vi "Uncaging Dual.vi"() -> ()   [LabVIEW 2012]
uses:
  Custom Controls and Typedefs/Calibrate_Button.ctl
  Custom Controls and Typedefs/SciScan System Information Cluster.ctl
  <vilib>/Utility/miscctls.llb/LVRowAndColumnTypeDef.ctl
  Custom Controls and Typedefs/LineScan settings Status.ctl
  Custom Controls and Typedefs/LineScan Image Status.ctl
  <vilib>/vision/Image Controls.llb/IMAQ Image.ctl
  <vilib>/Utility/miscctls.llb/LVRowAndColumnUnsignedTypeDef.ctl
  modules/hyperscope modules/hyperscope subVIs/Timebase and Trigger Routing.ctl
  Custom Controls/Image Types.ctl
  Custom Controls/scan mode main settings tab.ctl
  Custom Controls/MAIN Image panel reso tab Control type def.ctl
  Custom Controls/MAIN Image panel tab Control type def.ctl
  Custom Controls and Typedefs/SamplingRatesCluster.ctl
  Custom Controls and Typedefs/GroupParameters_Cluster.ctl
  Custom Controls and Typedefs/TriggerParameters_Cluster.ctl
  Custom Controls and Typedefs/UncageType.ctl
  GFG/GFG Translator Wrapper/GFGTranslator_Action.ctl
  GFG/GFG Translator Wrapper/GFGTranslator_Datatype.ctl
  GFG/GFG Translator Wrapper/GFGTranslator_errors.ctl
  GFG/GFGbooleanGet.vi
  GFG/GFGstringGet.vi
  save ROI.vi
  <vilib>/Utility/config.llb/Read Key (String).vi
  Global Variable_Waveforms.vi
  GFG/GFGfpRefGet.vi
  GFG/GFGpathGet.vi
  <vilib>/Utility/file.llb/Read From Spreadsheet File (string).vi
  GFG/GFG library.lvlib
  <vilib>/Utility/config.llb/NI_LVConfig.lvlib
panel:
  in  "Stimulation Protocol":enum32{"Protocol Editor", "Waveforms"}(tab)
  in  "Protocol Editor":i32[](listbox)
  in  "Enable/Disable All":bool=TRUE
  in  "Delete":bool
  in  "Reverse":bool
  in  "random":bool
  out "Waveform Graph":waveform(dbl)[](graph)
  out "StimModuleStatus":string caption="Status"
  in  "reset zoom_Photo-Stim_UI":bool
  out "Image1":T1(plugin-control)
  in  "Channel Selector":T2(tab)
  in  "Auto Update?":bool=TRUE
  out "Time for generating waveforms (ms)":u32
  in  "Update waveform and Timing":bool
  in  "Rep interval (s)":dbl=0.1 min=1.0 step=1.0
  in  "Pre-Stim Baseline":dbl
  in  "Pre-stim baseline (s)":bool
  in  "Group reps":dbl=1.0 min=1.0 step=1.0
  in  "Protocol Name":string="New_Stim_Protocol"
  in  "Load Stim Protocol":bool
  in  "Save Stim Protocol":bool
  in  "Columns":i32=6 min=1
  in  "Rows":i32=6 min=1
  in  "Y position":i32=128
  in  "X postition":i32=128
  in  "Grid spacing (µm)":dbl=10.0
  in  "GRID":bool
  in  "Spot repetitions":dbl=5.0 min=1.0 step=1.0
  in  "Stim duration (s)":dbl=0.0001 caption="(10u to 10m)" min=1e-05 max=0.01 step=1e-05 format="%#_6p"
  in  "Pre-stim settling time (s)":dbl=0.0008 caption="(800u to 1)" min=0.0008 max=1.0 format="%#_6p"
  in  "Stim interval (s)":dbl=0.00030000000000000003 caption="(300u to 1)" min=0.00030000000000000003 max=1.0 step=0.005 format="%#_6p"
  in  "Stim Power (%)":dbl(slide) min=0.0 max=100.0 step=0.1 scale=0.0..100.0
  out "Group Duration (s)":dbl
  in  "Uncage and Image":bool
  in  "Uncage ONLY":bool
  in  "stop":bool
  out "Total time (s)":dbl
  in  "Imaging Shutter":bool caption="Imaging Path Shutter"
  in  "Uncaging Shutter":bool caption="Stim Path Shutter"
  in  "Wait for external trigger":bool
  in  "Calibrate":T3
  # "General Stimulation Parameters"
  # "to zoom out press and hold Shift"
  # "Stimulation Protocol"
  # "Protocol Parameters"
  # "File Operations"
  # "Grid Parameters"
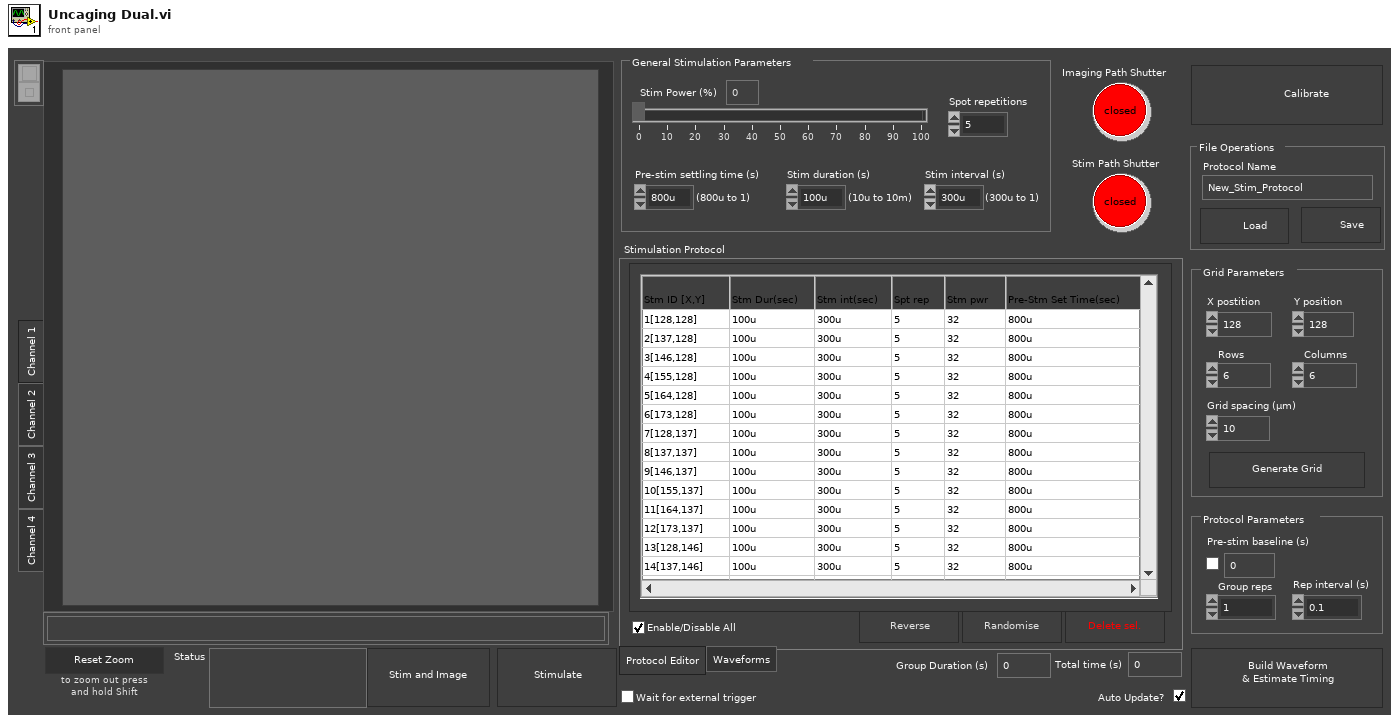
[diagram p1: front panel]
types:
  T1 = typedef "IMAQ Image.ctl" = refnum<image>
  T2 = enum32{"Channel 1", "Channel 2", "Channel 3", "Channel 4"}
  T3 = typedef "Calibrate_Button.ctl" = bool
  T4 = typedef "LineScan Image Status.ctl" = enum16{"not a LineScan image", "LineScan  image"}
  T5 = typedef "LineScan settings Status.ctl" = enum16{"not Linescan Settings", "LineScan Settings"}
  T6 = typedef "LVRowAndColumnTypeDef.ctl" = cluster{"Row":i32, "Column":i32}
  T7 = typedef "SciScan System Information Cluster.ctl" = cluster{"Scanner Type":string, "Is it Hyperscope?":bool, "Hyperscope (DAQ) type":string}
  T8 = enum16{"Init all tabs to a color", "Change specific tabs"}
  T9 = typedef "Image Type" = u32
  T10 = cluster{"ROI name":string, "pixel coordinates":cluster{"x":i32, "y":i32}}[]
  T11 = typedef "LVRowAndColumnUnsignedTypeDef.ctl" = cluster{"Row":u32, "Column":u32}
  T12 = enum8{"Enabled", "Disabled", "Disabled and Grayed Out"}
  T13 = typedef "NI_LVConfig.lvlib/Config Data RefNum.ctl" = refnum<k1>
  T14 = cluster{"Left":i32, "Top":i32, "Right":i32, "Bottom":i32}
  T15 = typedef "Timebase and Trigger Routing.ctl" = enum16{"Connect", "Disconnect all", "Disconnect Trigger"}
  T16 = cluster{"ROI name":string, "pixel coordinates":cluster{"x":i32, "y":i32}}
  T17 = typedef "Image Types.ctl" = enum16{"Frame Scan", "Line Scan", "RGB Overlay", "ROI", "All Channels Frame"}
  T18 = typedef "scan mode main settings tab.ctl" = enum32{"2D frame", "2D line scan", "general settings", "Z Stack", "piezo"}
  T19 = cluster{"X- Offset (in pixels)":i32, "Y-Offset (in pixels)":i32}
  T20 = cluster{"X Grid Spacing (in metres)":dbl, "Y Grid Spacing (in metres)":dbl}
  T21 = cluster{"X FOV (in metres)":dbl, "Y FOV (in metres)":dbl}
  T22 = typedef "TriggerParameters_Cluster.ctl" = cluster{"Pre-stim Wait":bool, "Wait for external trigger":bool}
  T23 = typedef "GroupParameters_Cluster.ctl" = cluster{"Group repetitions":i32, "Repetition Interval":dbl, "Pre-stim baseline":dbl}
  T24 = typedef "UncageType.ctl" = enum16{"Uncage Only", "Uncage & Image"}
  T25 = typedef "GFGTranslator_errors.ctl" = enum16{"Success", "SciScan Not Running", "No Get Method for Selected Datatype", "No Set Method for Selected Datatype", "Variable Not Found", "Unexpected Datatype", "Data Out of Range"}
  T26 = typedef "GFGTranslator_Datatype.ctl" = enum16{"String", "Path (String)", "Numeric", "Boolean", "Set_BoolRef (use boolean data)", "Get_Variant", "Get_2DArray (I16)", "Get_Image_2DArray (I16)", "Get_Version (String)", "Get_All GFG variables (String)"}
  T27 = typedef "GFGTranslator_Action.ctl" = enum16{"Get", "Set"}
  T28 = cluster{"Desired Font (Application)":enum16{"User-specified Font", "Application Font", "System Font", "Dialog Font"}, "[User-specified Font]":cluster{"Font Name":string, "Size":i16, "Strikeout?":bool, "Italic?":bool, "Underline?":bool, "Outline?":bool, "Shadow?":bool, "Bold?":bool, "Rotation Angle":dbl}, "Horizontal Alignment":i16, "Vertical Alignment":i16}
  T29 = enum32{"Invalid", "Standard", "Closed", "Hidden", "Minimized", "Maximized"}
  T30 = typedef "ROI Descriptor" = cluster{"Global Rectangle":i32[], "Contours":cluster{"ID":enum32{"External", "Internal"}, "Type":u32, "Coordinates":i32[]}[]}
  T31 = enum32{"Channel 1", "Channel 2", "Channel 3", "Channel 4"}[]
  T32 = typedef "MAIN Image panel reso tab Control type def.ctl" = enum32{"Channel 1", "Channel 2", "Channel 3", "Channel 4", "Channel 5", "all channels", "RGB overlay", "ROI", "arbitrary line scan"}
  T33 = typedef "MAIN Image panel tab Control type def.ctl" = enum32{"Channel 1", "Channel 2", "Channel 3", "Channel 4", "all channels", "RGB overlay", "ROI", "arbitrary line scan"}
  T34 = typedef "LVPoint32TypeDef.ctl" = cluster{"Horizontal":i32, "Vertical":i32}
  T35 = cluster{string, cluster{"X- Offset (in pixels)":i32, "Y-Offset (in pixels)":i32}}
  T36 = typedef "SamplingRatesCluster.ctl" = cluster{"AO samp rate_XY (samples/s)":dbl, "AO samp rate_Pockels (samples/s)":dbl, "DO samp rate_Gate (samples/s)":dbl}
  T37 = typedef "Stim Waveform Parameters.ctl" = cluster{"Stim Interval (Seconds)":dbl, "Pre-Stim Settling Time (Seconds)":dbl, "Stim Duration (Seconds)":dbl, "Spot Repetitions":i32, "Laser Power (%)":dbl, "XY Voltages":cluster{"X_Voltage (Volts)":dbl, "Y_Voltage (Volts)":dbl}, "Gate response lead (seconds)":dbl, "Gate response trail (seconds)":dbl}
  T38 = cluster{"WaveformChartRef":refnum<vi>, "DigitalRef":refnum<vi>, "ArrayRef":refnum<vi>, "TabControlRef":refnum<vi>, "EnumRef":refnum<vi>, "RingRef":refnum<vi>, "BooleanRef":refnum<vi>, "KnobRef":refnum<vi>, "SlideRef":refnum<vi>, "PathRef":refnum<vi>, "StringRef":refnum<vi>, "ComboBox":refnum<vi>, "WaveformGraphRef":refnum<vi>}
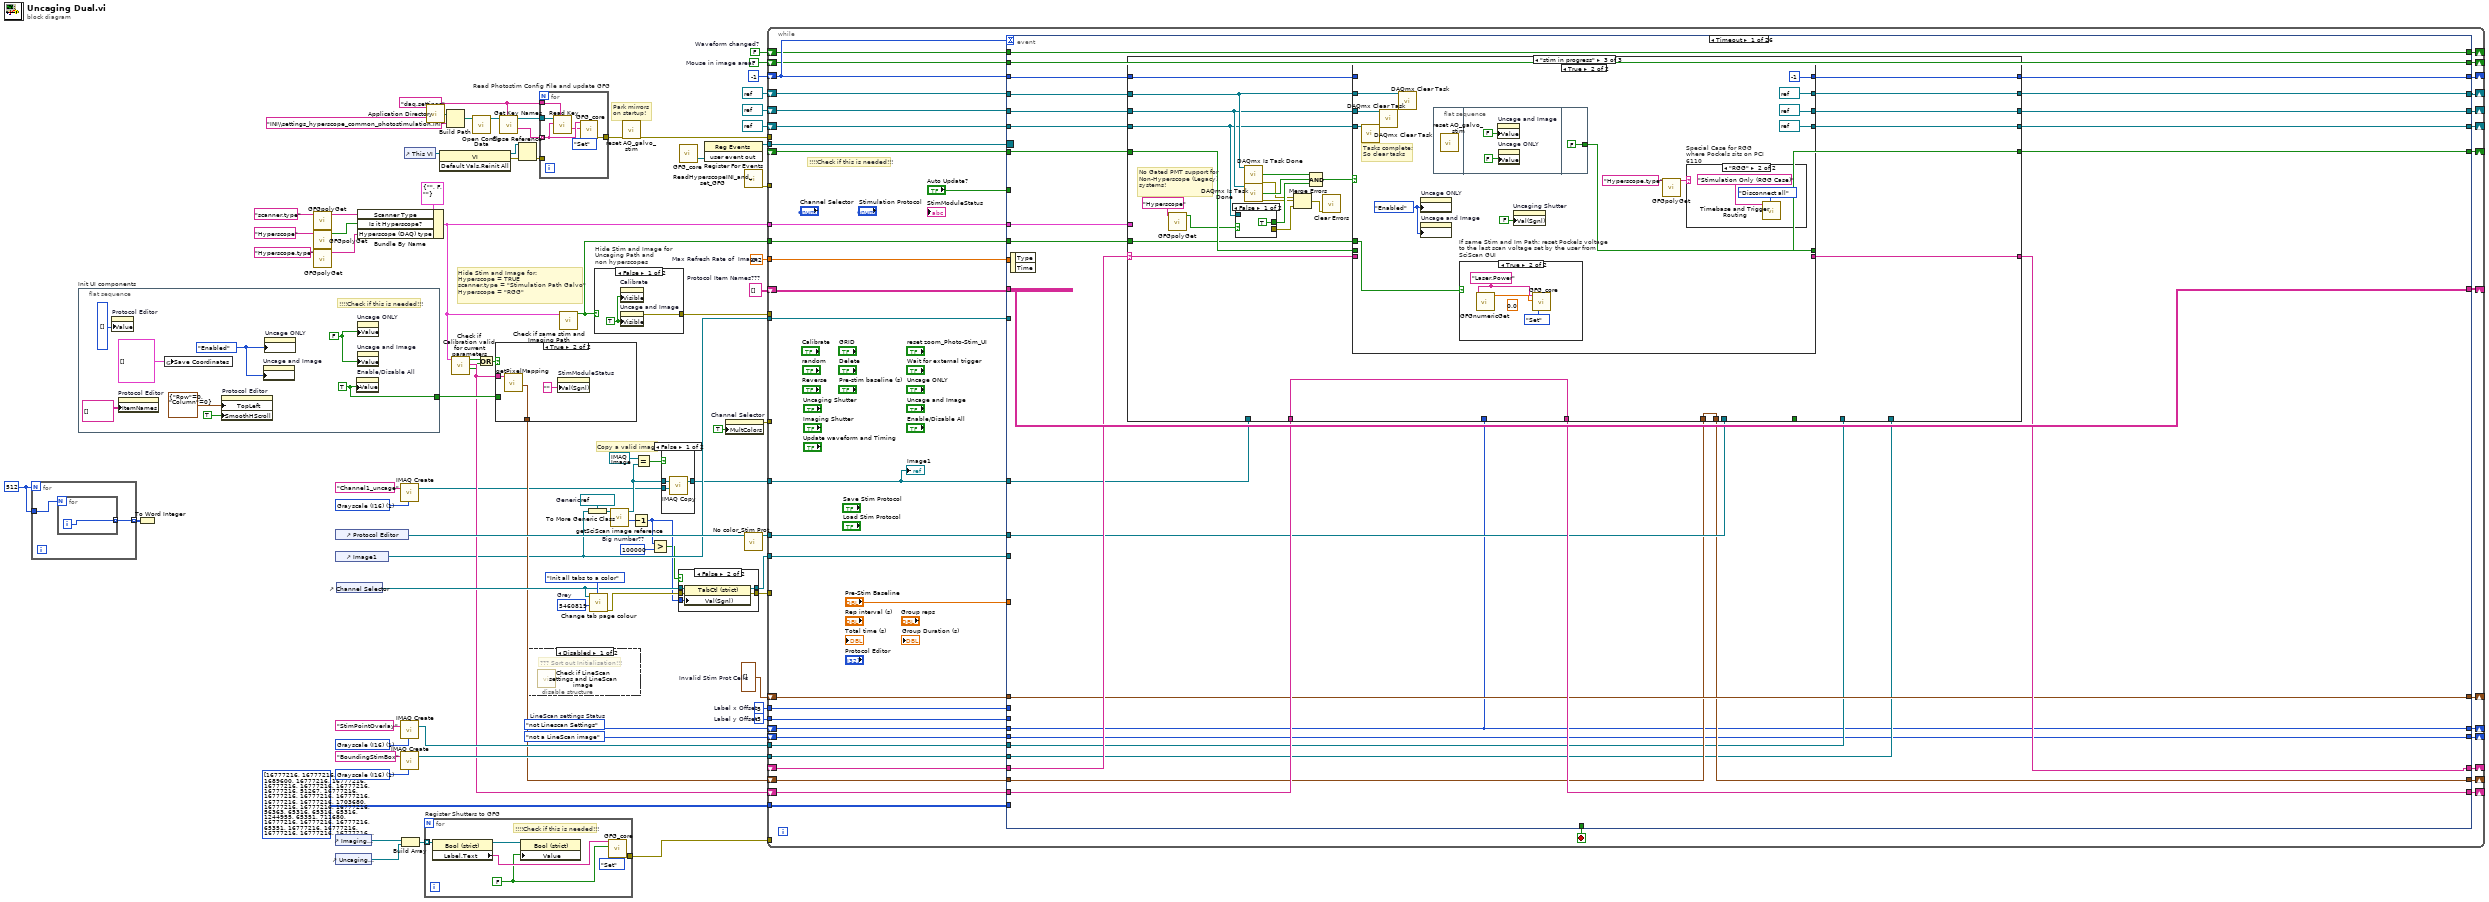
[diagram p0: block diagram]
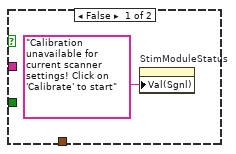
[diagram p5: hidden frame]
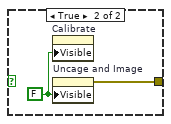
[diagram p6: hidden frame]
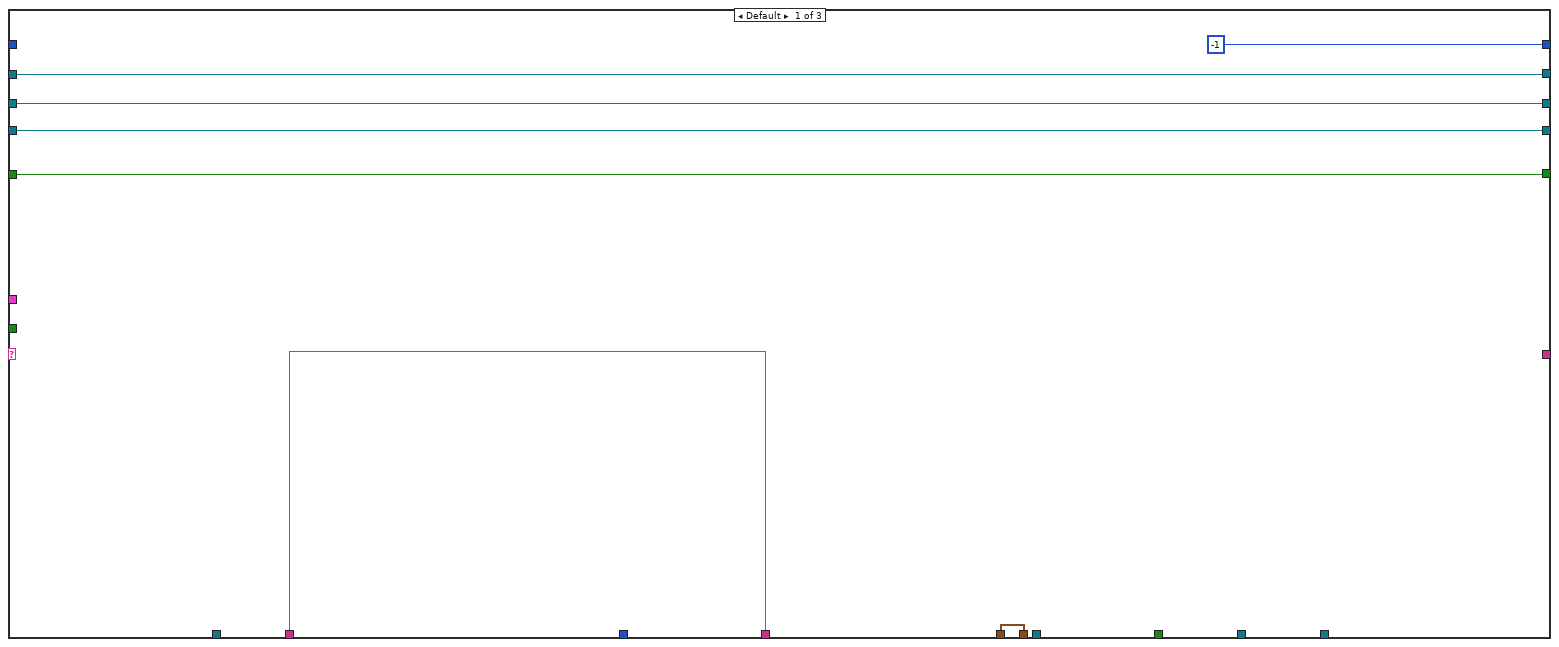
[diagram p7: hidden frame]
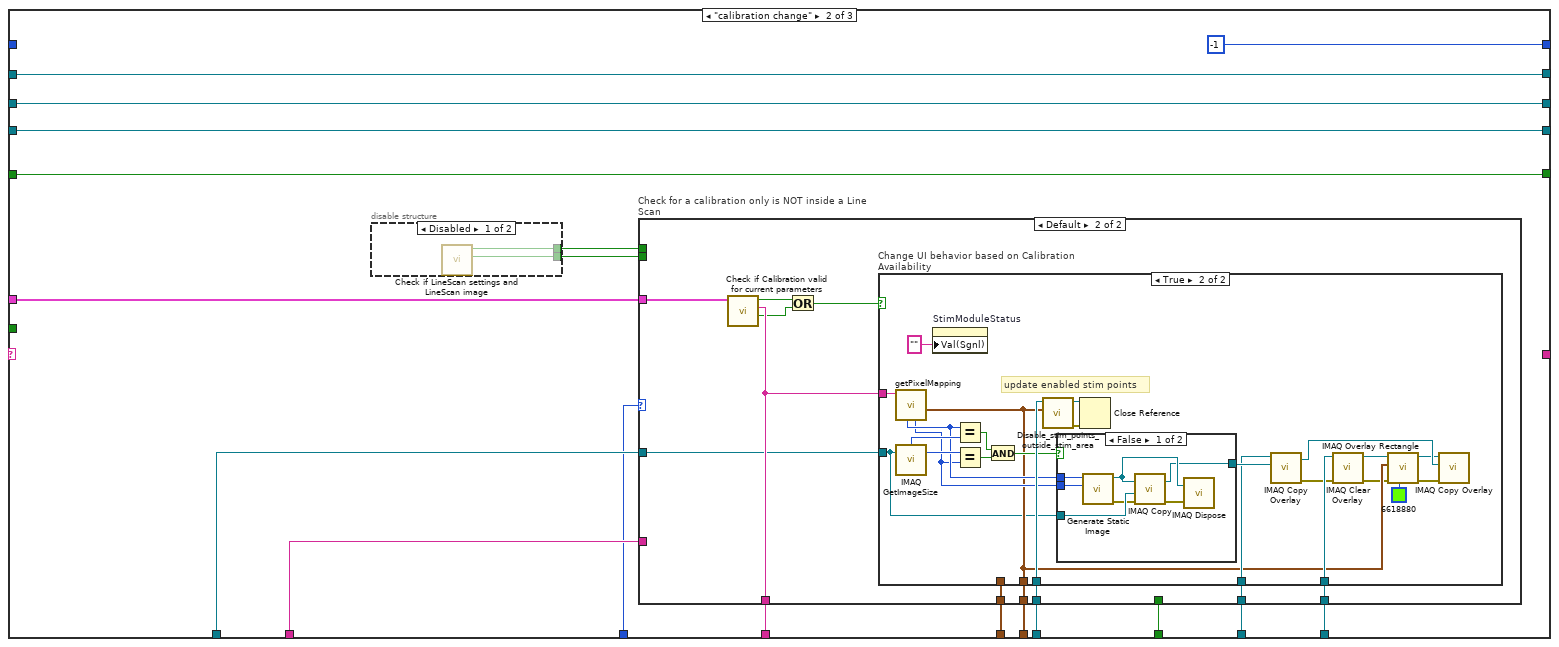
[diagram p8: hidden frame]
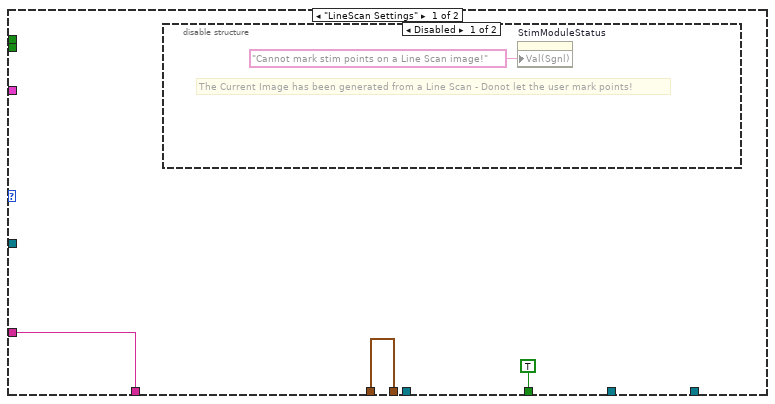
[diagram p10: hidden frame]
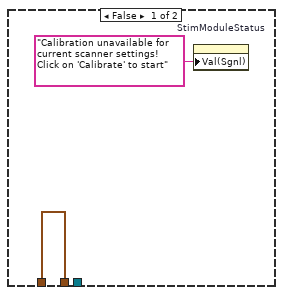
[diagram p12: hidden frame]
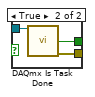
[diagram p14: hidden frame]
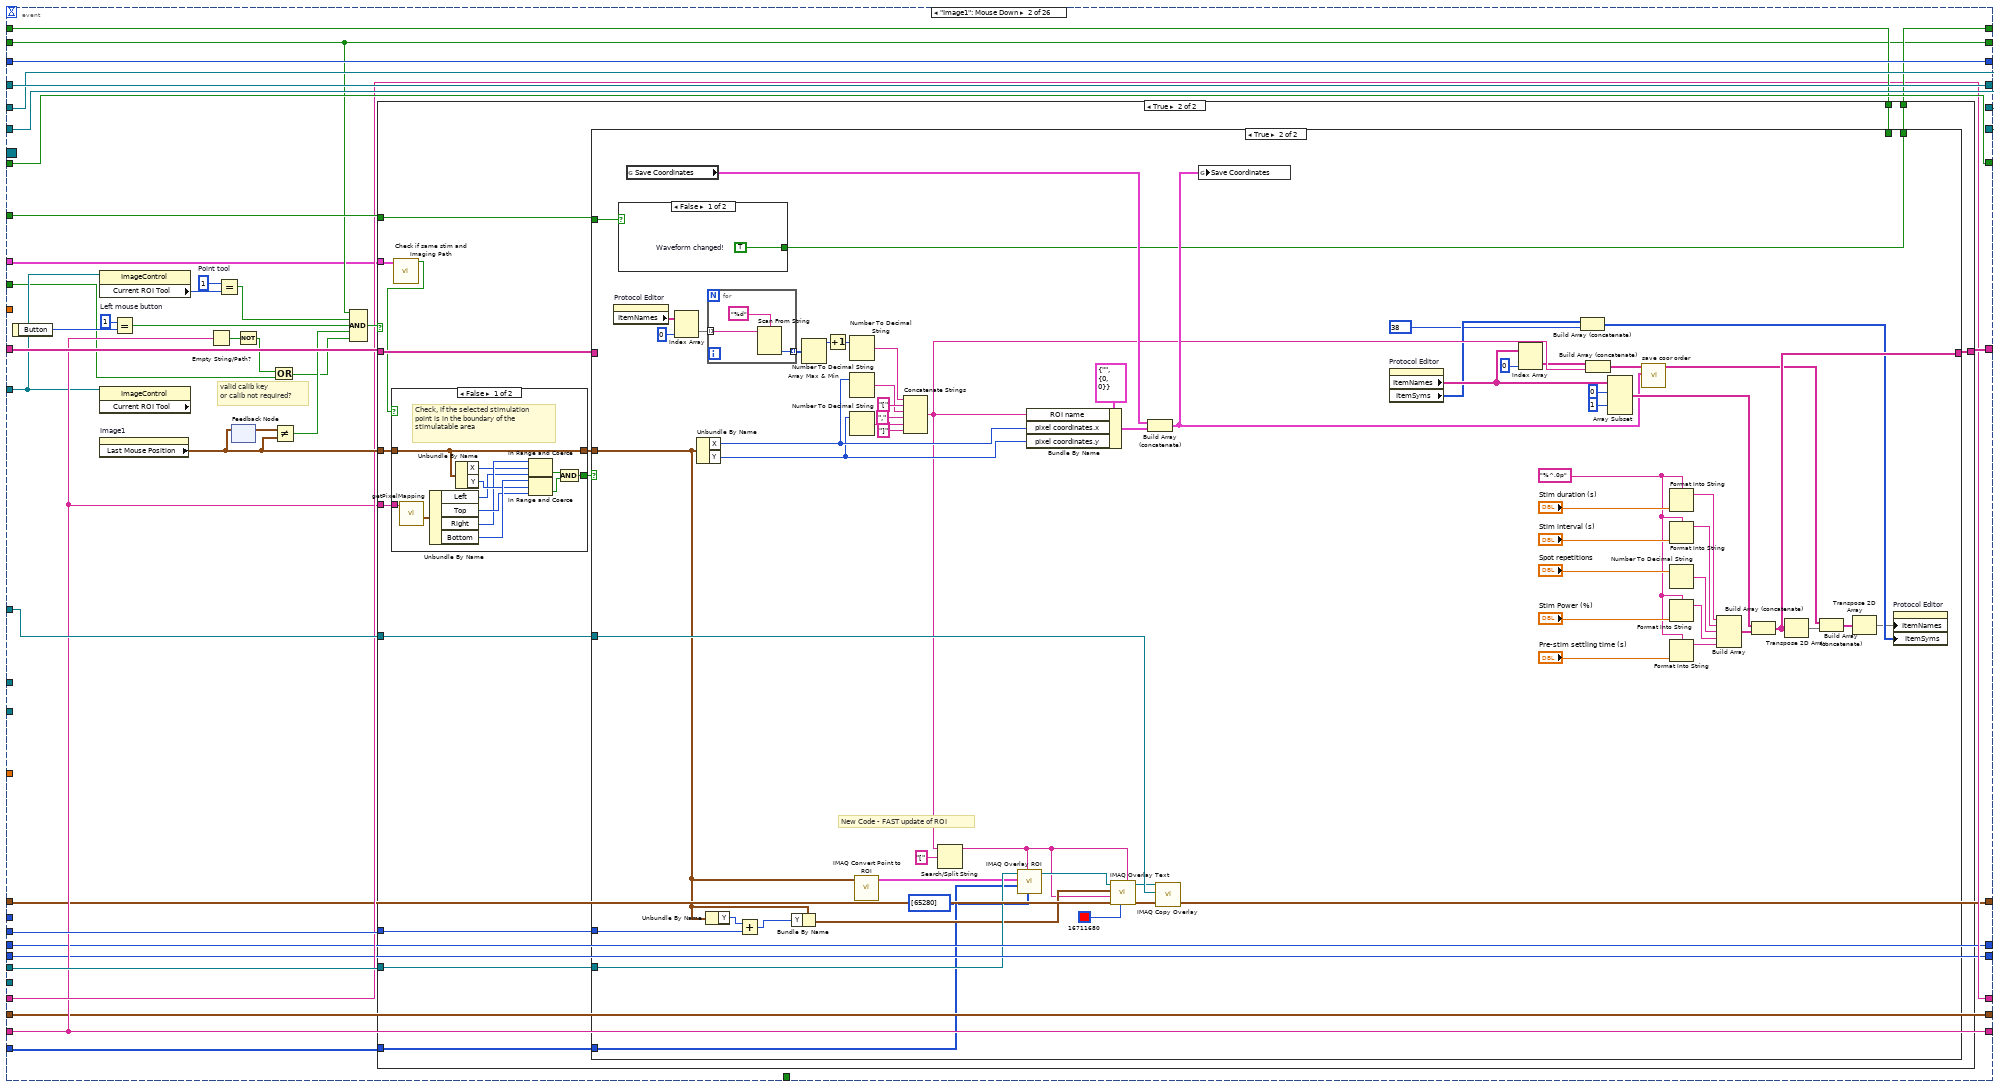
[diagram p18: hidden frame]
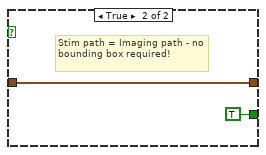
[diagram p20: hidden frame]
diagram:
  w7 = refnum<vi> refnum  # Generic
  w10 = 512
  w14 = u32 100000  # Big number??
  w17 = LineScan_settings_Status."not Linescan Settings"  # LineScan settings Status
  w22 = T6[] []  # Invalid Stim Prot Cells
  w35 = 5460819  # Grey
  w41 = T9 1 items=["Grayscale (U8)", "Grayscale (I16)", "Grayscale (SGL)", "Complex (CSG)", "RGB (U32)", "HSL (U32)", "RGB (U64)", "Grayscale (U16)"] ("Image Type")
  w43 = FALSE  # Mouse in image area?
  w54 = FALSE  # Waveform changed?
  w59 = "daq.settings" ("section")
  w63 = -5  # Label x Offset
  w64 = -5  # Label y Offset
  w67 = T9 1 items=["Grayscale (U8)", "Grayscale (I16)", "Grayscale (SGL)", "Complex (CSG)", "RGB (U32)", "HSL (U32)", "RGB (U64)", "Grayscale (U16)"] ("Image Type")
  w70 = 0.2  # Max Refresh Rate of  Image
  w72 = T9 1 items=["Grayscale (U8)", "Grayscale (I16)", "Grayscale (SGL)", "Complex (CSG)", "RGB (U32)", "HSL (U32)", "RGB (U64)", "Grayscale (U16)"] ("Image Type")
  w82 = string[][] []  # Protocol Item Names???
  # "Copy a valid image"
  # "Park mirrors\non startup!"
  # "Hide Stim and Image for:\nHyperscope = TRUE    \nscanner.type = \"Stimulation Path Galvo\"\nHyperscope = \"RGG\""
  n1 = for {
    N: w10 -> [_]
    tunnel: w10 -> [w83]
    tunnel: [w84] -> w9 mode=indexing
    n2 = for {
      N: w83 -> [_]
      tunnel: [w85] -> w84 mode=indexing
      i -> [w85]
    }
  }
  n3 = flat-sequence "Init UI components" {
    tunnel: [w86] -> w24
    frame #0 {
      w92 = T12."Enabled" ("Disabled")
      w93 = FALSE ("Boolean")
      w86 = TRUE ("Deselect all")
      # "!!!!Check if this is needed!!!"
      n4 = property on="Protocol Editor" class="MCListbox (strict)"("Value"=i32[] [] ("Stimulation Protocol")) -> ()  [unwired: 2 in, 2 out]
      n5 = property on="Protocol Editor" class="MCListbox (strict)"("ItemNames"=string[][] [] ("Item Names")) -> ()  [unwired: 2 in, 2 out]
      n6 = global write "save ROI.vi" "Save Coordinates"(T10 [] ("Save Coordinates")) -> ()
      n7 = property on="Protocol Editor" class="MCListbox (strict)"("TopLeft"=T11 {"Row"=0, "Column"=0} ("Top Left Visible Cell"), "SmoothHScroll"=TRUE ("Smooth Horizontal Scrolling")) -> ()  [unwired: 2 in, 2 out]
      n8 = property on="Uncage and Image" class="Bool (strict)"("DisabledEnum"=w92) -> ()  [unwired: 2 in, 2 out]
      n9 = property on="Uncage ONLY" class="Bool (strict)"("DisabledEnum"=w92) -> ()  [unwired: 2 in, 2 out]
      n10 = property on="Enable/Disable All" class="Bool (strict)"("Value"=w86) -> ()  [unwired: 2 in, 2 out]
      n11 = property on="Uncage ONLY" class="Bool (strict)"("Value"=w93) -> ()  [unwired: 2 in, 2 out]
      n12 = property on="Uncage and Image" class="Bool (strict)"("Value"=w93) -> ()  [unwired: 2 in, 2 out]
    }
  }
  n13 = To Word Integer(number=w9) -> ()  [unwired: 1 out]
  n14 = call-poly "GFGpolyGet.vi"("Variable Name in"="scanner.type") -> ("String"=w29:string)  [unwired: 9 in, 1 out]
  n15 = call-poly "GFGpolyGet.vi"("Variable Name in"="Hyperscope") -> ("Boolean Value OUT"=w28:bool)  [unwired: 9 in, 1 out]
  n16 = call-poly "GFGpolyGet.vi"("Variable Name in"="Hyperscope.type") -> ("String"=w27:string)  [unwired: 9 in, 1 out]
  n17 = control-ref of="Protocol Editor"() -> (w71:refnum<vi>)
  n18 = control-ref of="Image1"() -> (w18:refnum<vi>)
  n19 = control-ref of="Imaging Shutter"() -> (w79:refnum<vi>)
  n20 = control-ref of="Uncaging Shutter"() -> (w78:refnum<vi>)
  n21 = control-ref of="Channel Selector"() -> (w32:refnum<vi>)
  n22 = Bundle By Name(cluster=T7 {"Scanner Type"="", "Is it Hyperscope?"=FALSE, "Hyperscope (DAQ) type"=""} ("System Information Cluster"), "Scanner Type"=w29, "Is it Hyperscope?"=w28, "Hyperscope (DAQ) type"=w27) -> (w25:T7)
  n23 = call "IMAQ Create"("Image Name"="Channel1_uncage", "Image Type"=w72) -> ("New Image"=w2:T1)  [unwired: 3 in, 1 out]
  n24 = call "IMAQ Create"("Image Name"="StimPointOverlay", "Image Type"=w67) -> ("New Image"=w40:T1)  [unwired: 3 in, 1 out]
  n25 = call "IMAQ Create"("Image Name"="BoundingStimBox", "Image Type"=w41) -> ("New Image"=w39:T1)  [unwired: 3 in, 1 out]
  n26 = Build Array(w79, w78) -> (w77:refnum<vi>[])
  n27 = control-ref of="This VI"() -> (w53:refnum<vi>)
  n28 = for "Register Shutters to GFG" {
    tunnel: w77 -> [w99] mode=indexing
    tunnel: [w94] -> w76
    w95 = FALSE ("Value")
    # "!!!!Check if this is needed!!!"
    n29 = property class="Bool (strict)"(reference=w99) -> (reference out=w98:refnum<vi>, "Label.Text"=w96:string)  [unwired: 1 in, 1 out]
    n30 = property class="Bool (strict)"(reference=w98, "Value"=w95) -> ()  [unwired: 1 in, 2 out]
    n31 = call "GFG_core.vi"("Variable Name in"=w96, "Variant in"=w95, "Action"=enum16{"Init", "Set", "Get", "Clear"}."Set") -> ("error out"=w94:errorcluster)  [unwired: 10 in, 6 out]
  }
  n32 = call <vilib>:"Application Directory.vi"() -> ("Application Directory"=w62:path)
  n33 = invoke class="VI" method="Default Vals.Reinit All"(reference=w53) -> (reference out=w51:refnum<vi>, error out=w52:errorcluster)  [unwired: 2 in, 1 out]
  n34 = Build Path(base path=w62, name or relative path="INI\\settings_hyperscope_common_photostimulation.ini") -> (appended path=w60:path)
  n35 = call "Check if Calibration valid for current parameters.vi"("System Information Cluster"=w25) -> ("Calibration Not Required?"=w11:bool, "Current Calibration Key"=w20:string, "Calibration Valid?"=w23:bool)  [unwired: 8 in]
  n36 = call <vilib>:"Open Config Data.vi"("configuration file path"=w60) -> ("refnum"=w58:T13)  [unwired: 8 in, 2 out]
  n37 = Or(x=w23, y=w11) -> (x .or. y?=w12:bool)
  n38 = case shown="True" w12 {
    tunnel: w24 -> [_ _]
    tunnel: w20 -> [_ w102]
    tunnel: [_ w101] -> w19
    frame False {
      n39 = property on="StimModuleStatus" class="Str"("Val(Sgnl)"="Calibration unavailable for current scanner settings! Click on 'Calibrate' to start" ("Variable Name in")) -> ()  [unwired: 2 in, 2 out]
    }
    frame True {
      n40 = call "getPixelMapping.vi"("Key String IN"=w102) -> ("Rectangle"=w101:T14)  [unwired: 5 in, 5 out]
      n41 = property on="StimModuleStatus" class="Str"("Val(Sgnl)"="" ("Variable Name in")) -> ()  [unwired: 2 in, 2 out]
    }
  }
  n42 = call <vilib>:"Get Key Names.vi"("section"=w59, "refnum"=w58) -> ("key names"=w56:string[], "refnum out"=w57:T13)  [unwired: 6 in, 2 out]
  n43 = Close Reference(reference=w51, error in (no error)=w52) -> (error out=w50:errorcluster)
  n44 = disable-structure shown="Disabled" {
    frame Disabled {
      # "??? Sort out Initialisation!!!"
      n45 = call "Check if LineScan settings and LineScan image.vi"() -> ()  [unwired: 10 in, 2 out]
    }
    frame Enabled {
    }
  }
  n46 = for "Read Photostim Config File and update GFG" {
    tunnel: w59 -> [w109]
    tunnel: w57 -> [w108]
    tunnel: w56 -> [w106] mode=indexing
    tunnel: [w104] -> w38
    tunnel: w50 -> [_]
    n47 = call-poly <vilib>:"Read Key.vi"("section"=w109, "key"=w106, "refnum"=w108) -> ("value"=w105:string)  [unwired: 5 in, 3 out]
    n48 = call "GFG_core.vi"("Variable Name in"=w106, "Variant in"=w105, "Action"=enum16{"Init", "Set", "Get", "Clear"}."Set") -> ("error out"=w104:errorcluster)  [unwired: 10 in, 6 out]
  }
  n49 = call "Check if same stim and Imaging Path.vi"("System Information Cluster"=w25) -> ("Boolean"=w26:bool)  [unwired: 10 in]
  n50 = To More Generic Class(target class=w7, reference=w18) -> (generic class reference=w8:refnum<vi>)
  n51 = call "Change tab page colour.vi"("Action"=T8."Init all tabs to a color", "New Colour"=w35, "TabControl in"=w32) -> ("error out"=w34:errorcluster)  [unwired: 8 in]
  n52 = case "Hide Stim and Image for \nUncaging Path and \nnon hyperscopes" shown="False" w26 {
    tunnel: [w111 w113] -> w47
    frame False {
      w110 = TRUE ("Visible")
      n53 = property on="Calibrate" class="Bool"("Visible"=w110) -> ()  [unwired: 2 in, 2 out]
      n54 = property on="Uncage and Image" class="Bool (strict)"("Visible"=w110) -> (error out=w111:errorcluster)  [unwired: 2 in, 1 out]
    }
    frame True {
      w112 = FALSE ("Visible")
      n55 = property on="Calibrate" class="Bool"("Visible"=w112) -> ()  [unwired: 2 in, 2 out]
      n56 = property on="Uncage and Image" class="Bool (strict)"("Visible"=w112) -> (error out=w113:errorcluster)  [unwired: 2 in, 1 out]
    }
  }
  n57 = call "getSciScan image reference.vi"("Image Refnum (Generic)"=w8) -> ("Channel Number"=w6:u32, "Current Image"=w4:T1)  [unwired: 6 in, 3 out]
  n58 = call "reset AO_galvo_stim.vi"("error in (no error)"=w38) -> ("error out"=w37:errorcluster)  [unwired: 10 in]
  n59 = Decrement(x=w6) -> (x-1=w15:u32)
  n60 = Equal?(x=T1 refnum, y=w4) -> (x = y?=w3:bool)
  n61 = Greater?(x=w15, y=w14) -> (0:w13:bool)
  n62 = case shown="False" w3 {
    tunnel: [w116 w117] -> w1
    tunnel: w2 -> [w115 w117]
    tunnel: w4 -> [w114 _]
    frame False {
      n63 = call "IMAQ Copy"("Image Dst"=w115, "Image Src"=w114) -> ("Image Dst Out"=w116:T1)  [unwired: 4 in, 1 out]
    }
    frame True {
    }
  }
  n64 = case shown="False" w13 {
    tunnel: w34 -> [w118 w124]
    tunnel: [w118 w123] -> w33
    tunnel: w32 -> [w119 w122]
    tunnel: [w119 w121] -> w31
    tunnel: w15 -> [_ w120]
    frame True {
    }
    frame False {
      n65 = property class="TabCtl (strict)"(reference=w122, error in=w124, "Val(Sgnl)"=w120) -> (reference out=w121:refnum<vi>, error out=w123:errorcluster)
    }
  }
  n66 = call "GFG_core.vi"() -> ("user event out"=w75:refnum<user-event>)  [unwired: 13 in, 6 out]
  n67 = register-events(w75) -> (reference out=w74:refnum<event-registration>)  [unwired: 2 in, 1 out]
  n68 = property on="Channel Selector" class="TabCtl (strict)"("MultColors"=TRUE ("Allow Multiple Colors")) -> (error out=w44:errorcluster)  [unwired: 2 in, 1 out]
  n69 = call "ReadHyperscopeINI_and_set_GFG.vi"() -> ("error out"=w81:errorcluster)  [unwired: 11 in]
  n70 = call "No color_Stim Prot.vi"("Protocol Editor reference IN"=w71) -> ("Protocol Editor reference OUT"=w21:refnum<vi>)  [unwired: 9 in, 1 out]
  n71 = while {
    shift-right: [w167] -> _
    shift-left: w82 -> [w168]
    tunnel: w81 -> [_]
    shift-right: [w165] -> _
    shift-left: refnum<k21> refnum ("XY Mirror voltage Task OUT") -> [w163]
    shift-right: [w164] -> _
    shift-left: refnum<k21> refnum ("Pockels and Piezo Task OUT") -> [w162]
    shift-right: [w160] -> _
    shift-left: -1 -> [w161]
    tunnel: w76 -> [_]
    tunnel: w74 -> [w159]
    tunnel: w1 -> [w140]
    tunnel: w21 -> [w157]
    tunnel: w70 -> [w156]
    tunnel: w40 -> [w155]
    tunnel: u32[][] [[16777216, 16777216, 16777216, 1689600, 16777216, 16777216, 16777216], [16777216, 16777216, 16777216, 51267, 16777216, 16777216, 16777216], [16777216, 16777216, 16777216, 1703680, 16777216, 16777216, 16777216], [56363, 65316, 65316, 65316, 1244955, 65351, 711680], [16777216, 16777216, 16777216, 65351, 16777216, 16777216, 16777216], [16777216, 16777216, 16777216, 1244955, 16777216, 16777216, 16777216], [16777216, 16777216, 16777216, 1244955, 16777216, 16777216, 16777216]] ("Point Symbol") -> [w154]
    tunnel: w64 -> [w153]
    tunnel: w63 -> [w152]
    shift-right: [w150] -> _
    shift-left: _ -> [w149]
    shift-right: [w148] -> _
    shift-left: refnum<k21> refnum ("Pockels and Piezo Task OUT") -> [w147]
    shift-right: [w145] -> _
    shift-left: w54 -> [w146]
    tunnel: w47 -> [_]
    tunnel: w44 -> [_]
    tunnel: w31 -> [w144]
    tunnel: w33 -> [_]
    shift-right: [w141] -> _
    shift-left: w43 -> [w142]
    tunnel: w39 -> [w143]
    tunnel: w37 -> [_]
    tunnel: w25 -> [w139]
    tunnel: w26 -> [w138]
    shift-right: [w136] -> _
    shift-left: _ -> [w137]
    shift-right: [w134] -> _
    shift-left: w20 -> [w135]
    shift-right: [w132] -> _
    shift-left: w22 -> [w133]
    tunnel: w18 -> [w131]
    shift-right: [w129] -> _
    shift-left: w19 -> [w130]
    shift-right: [w127] -> _
    shift-left: w17 -> [w128]
    shift-right: [w125] -> _
    shift-left: LineScan_Image_Status."not a LineScan image" -> [w126]
    stop <- w166 stop-if-true
    # "!!!!Check if this is needed!!!"
    n72 = event shown="[0] Timeout" {
      selector: w159 -> [_ _ _ _ _ _ _ _ _ _ _ _ _ _ _ _ _ _ _ _ _ _ _ _ _ _]
      dyn-events: _ -> [_ _ _ _ _ _ _ _ _ _ _ _ _ _ _ _ _ _ _ _ _ _ _ _ _ _]
      timeout: w161 -> [_ _ _ _ _ _ _ _ _ _ _ _ _ _ _ _ _ _ _ _ _ _ _ _ _ _]
      tunnel: w168 -> [w194 w364 w482 w496 w512 w536 w839 w864 w910 w987 w1071 w1128 w1225 w1352 w1388 w1402 w1550 w1607 w1739 w1774 w1840 w1889 w2008 w2026 w2040 w2063]
      tunnel: [w194 w365 w482 w496 w512 w536 w839 w864 w910 w987 w1071 w1128 w1225 w1352 w1388 w1402 w1550 w1607 w1739 w1774 w1840 w1889 w2008 w2026 w2040 w2063] -> w167
      tunnel: [_ _ _ _ _ w534 _ _ _ _ _ _ _ _ _ _ _ _ _ _ _ _ _ _ "stop" _] -> w166
      tunnel: [w195 w363 w481 w495 w511 w541 w838 w863 w913 w986 w1074 w1132 w1219 w1351 w1387 w1409 w1555 w1616 w1742 w1777 w1843 w1893 w2011 w2025 w2043 w2062] -> w165
      tunnel: [w196 w362 w480 w494 w510 w540 w837 w862 w912 w985 w1073 w1131 w1218 w1350 w1386 w1408 w1554 w1615 w1741 w1776 w1842 w1892 w2010 w2024 w2042 w2061] -> w164
      tunnel: w163 -> [w193 w363 w481 w495 w511 w541 w838 w863 w913 w986 w1074 w1132 w1219 w1351 w1387 w1405 w1555 w1616 w1742 w1777 w1843 w1893 w2011 w2025 w2043 w2062]
      tunnel: w162 -> [w189 w362 w480 w494 w510 w540 w837 w862 w912 w985 w1073 w1131 w1218 w1350 w1386 w1404 w1554 w1615 w1741 w1776 w1842 w1892 w2010 w2024 w2042 w2061]
      tunnel: w161 -> [w185 w361 w479 w493 w509 w523 w836 w861 w911 w984 w1072 w1130 w1226 w1349 w1385 w1406 w1553 w1614 w1740 w1775 w1841 w1891 w2009 w2023 w2041 w2060]
      tunnel: [w184 w361 w479 w493 w509 w522 w836 w861 w911 w984 w1072 w1130 w1227 w1349 w1385 w1407 w1553 w1614 w1740 w1775 w1841 w1891 w2009 w2023 w2041 w2060] -> w160
      tunnel: w140 -> [w178 w360 _ _ _ w537 _ _ _ _ _ w1127 _ _ _ _ w1549 w1597 _ _ _ w1888 _ _ _ _]
      tunnel: w131 -> [_ w334 _ _ w505 w535 _ _ _ _ _ _ _ _ _ _ _ _ _ _ _ _ _ _ _ _]
      tunnel: "Pre-Stim Baseline" -> [_ _ _ _ _ _ _ _ _ _ _ _ w1224 _ _ _ _ _ _ _ _ _ _ _ _ _]
      tunnel: w157 -> [w176 _ _ _ _ _ _ _ w882 _ w1061 _ _ _ _ _ _ w1594 _ w1766 w1823 w1878 _ _ _ _]
      tunnel: w156 -> [_ _ _ _ _ w533 _ _ _ _ _ _ _ _ _ _ _ _ _ _ _ _ _ _ _ _]
      tunnel: w155 -> [w173 w359 _ _ _ w532 _ _ _ _ _ w1101 _ _ _ _ _ w1595 _ _ _ w1887 _ _ _ _]
      tunnel: w154 -> [_ w358 _ _ _ _ _ _ _ _ _ w1103 _ _ _ _ _ _ _ _ _ _ _ _ _ _]
      tunnel: w153 -> [_ w357 _ _ _ _ _ _ _ _ _ w1098 _ _ _ _ _ _ _ _ _ _ _ _ _ _]
      tunnel: w152 -> [_ _ _ _ _ _ _ _ _ _ _ w1099 _ _ _ _ _ _ _ _ _ _ _ _ _ _]
      tunnel: "Auto Update?" -> [_ w350 _ _ _ _ _ _ w906 w970 w1067 w1095 _ _ _ _ _ _ _ w1771 w1837 w1882 _ w2020 _ _]
      tunnel: [w190 w356 w478 w492 w508 w531 w833 w860 w909 w983 w1070 w1097 w1223 w1348 w1384 w1401 w1548 w1606 w1735 w1773 w1839 w1886 w1997 w2022 w2039 w2054] -> w150
      tunnel: w149 -> [w186 w356 w478 w492 w508 w531 w833 w860 w909 w983 w1070 w1097 w1223 w1348 w1384 w1400 w1548 w1606 w1735 w1773 w1839 w1886 w1997 w2022 w2039 w2054]
      tunnel: [w192 w355 w477 w491 w507 w530 w829 w859 w908 w982 w1069 w1096 w1222 w1347 w1383 w1399 w1547 w1605 w1732 w1772 w1838 w1885 w1996 w2021 w2038 w2053] -> w148
      tunnel: w147 -> [w188 w355 w477 w491 w507 w530 w829 w859 w908 w982 w1069 w1096 w1222 w1347 w1383 w1398 w1547 w1605 w1732 w1772 w1838 w1885 w1996 w2021 w2038 w2053]
      tunnel: w146 -> [w191 w354 w476 w490 w506 w529 w828 w858 w904 w969 _ _ w1220 w1346 w1382 w1397 w1546 w1604 w1731 _ _ w1883 w1995 _ w2037 w2052]
      tunnel: [w191 w353 w476 w490 w506 w529 w828 w858 w905 w968 w1066 w1094 w1221 w1346 w1382 w1397 w1546 w1604 w1731 w1770 w1836 w1884 w1995 w2019 w2037 w2052] -> w145
      tunnel: w144 -> [_ _ _ _ _ w527 _ w851 _ _ _ _ _ _ _ _ _ _ _ _ _ _ _ _ _ _]
      tunnel: w143 -> [w172 _ _ _ _ w526 _ _ _ _ _ w1083 _ _ _ _ _ w1596 _ _ _ _ _ _ _ _]
      tunnel: w142 -> [w187 w346 _ _ w503 w525 w827 w857 w907 w981 w1065 w1093 w1216 w1345 w1381 w1396 w1545 w1603 w1730 w1769 w1835 w1881 w1994 w2018 w2036 w2051]
      tunnel: [w187 w346 FALSE TRUE w503 w525 w827 w857 w907 w981 w1065 w1093 w1216 w1345 w1381 w1396 w1545 w1603 w1730 w1769 w1835 w1881 w1994 w2018 w2036 w2051] -> w141
      tunnel: w139 -> [w183 w329 _ _ _ w524 _ _ _ _ _ w1082 _ _ _ _ _ w1589 _ _ _ _ _ _ _ _]
      tunnel: w138 -> [w169 w330 _ _ _ _ _ _ _ _ _ _ w1211 w1333 _ w1389 _ _ _ _ _ _ _ _ _ _]
      tunnel: w137 -> [w182 w340 w474 w488 w502 w521 w826 w848 w903 w980 w1064 w1092 w1215 w1344 w1380 _ w1544 w1600 w1729 w1768 w1834 w1880 w1993 w2017 w2035 w2050]
      tunnel: [w181 w340 w474 w488 w502 w515 w826 w848 w903 w980 w1064 w1092 w1215 w1344 w1380 w1395 w1544 w1600 w1729 w1768 w1834 w1880 w1993 w2017 w2035 w2050] -> w136
      tunnel: w135 -> [w180 w338 w473 w487 w501 w520 w825 w847 w902 w979 w1063 w1085 w1209 w1339 w1379 w1394 w1543 w1590 w1728 w1767 w1833 w1879 w1992 w2016 w2034 w2049]
      tunnel: [w179 w338 w473 w487 w501 w520 w825 w847 w902 w979 w1063 w1085 w1209 w1339 w1379 w1394 w1543 w1590 w1728 w1767 w1833 w1879 w1992 w2016 w2034 w2049] -> w134
      tunnel: w133 -> [w177 w337 w472 w486 w500 w519 w824 w846 w901 w974 w1062 w1091 w1208 w1341 w1378 w1393 w1542 w1598 w1727 w1750 _ w1876 w1991 w2015 w2033 w2048]
      tunnel: [w177 w337 w472 w486 w500 w519 w824 w846 w901 w973 w1062 w1091 w1208 w1341 w1378 w1393 w1542 w1599 w1727 w1753 w1811 w1877 w1991 w2015 w2033 w2048] -> w132
      tunnel: w130 -> [w174 w336 w471 w485 w499 w518 w823 w845 w883 w967 w1052 w1090 w1207 w1337 w1377 w1392 w1541 w1593 w1726 w1748 w1810 w1875 w1990 w2014 w2032 w2047]
      tunnel: [w175 w336 w471 w485 w499 w518 w823 w845 w883 w967 w1052 w1090 w1207 w1337 w1377 w1392 w1541 w1593 w1726 w1748 w1810 w1875 w1990 w2014 w2032 w2047] -> w129
      tunnel: w128 -> [w170 w335 w470 w484 w498 w517 w822 w844 w881 w966 w1051 w1089 w1206 w1336 w1376 w1391 w1540 w1592 w1725 w1747 w1809 w1874 w1989 w2013 w2031 w2046]
      tunnel: [w170 w335 w470 w484 w498 w516 w822 w844 w881 w966 w1051 w1089 w1206 w1336 w1376 w1391 w1540 w1592 w1725 w1747 w1809 w1874 w1989 w2013 w2031 w2046] -> w127
      tunnel: w126 -> [w171 w333 w469 w483 w497 w514 w821 w843 w880 w965 w1050 w1088 w1205 w1335 w1375 w1390 w1539 w1591 w1724 w1746 w1808 w1873 w1988 w2012 w2030 w2045]
      tunnel: [w171 w333 w469 w483 w497 w513 w821 w843 w880 w965 w1050 w1088 w1205 w1335 w1375 w1390 w1539 w1591 w1724 w1746 w1808 w1873 w1988 w2012 w2030 w2045] -> w125
      event Timeout {
        n73 = event-data() -> ()  [unwired: 1 in, 2 out]
        n74 = case shown="\"stim in progress\"" w182 {
          selector: w182 -> [_ _ w279]
          tunnel: [w201 w219 w297] -> w196
          tunnel: [w200 w218 w296] -> w195
          tunnel: w193 -> [w200 w218 w295]
          tunnel: [w202 w220 w294] -> w192
          tunnel: [w203 w221 w293] -> w190
          tunnel: w189 -> [w201 w219 w292]
          tunnel: w188 -> [w202 w220 w291]
          tunnel: w186 -> [w203 w221 w286]
          tunnel: w185 -> [_ _ w285]
          tunnel: [-1 -1 w280] -> w184
          tunnel: w183 -> [_ w217 _]
          tunnel: [_ _ w278] -> w181
          tunnel: [w198 w214 w277] -> w179
          tunnel: w180 -> [w198 w208 w277]
          tunnel: w178 -> [_ w209 _]
          tunnel: w176 -> [_ w215 _]
          tunnel: [w197 w213 w276] -> w175
          tunnel: w174 -> [w197 w212 w276]
          tunnel: w173 -> [_ w211 _]
          tunnel: w172 -> [_ w210 _]
          tunnel: [_ w207 _] -> _
          tunnel: w170 -> [_ w204 _]
          tunnel: w169 -> [_ _ w275]
          frame Default {
          }
          frame "calibration change" {
            n75 = disable-structure shown="Disabled" {
              disable-tunnel: [w223 _] -> w206
              disable-tunnel: [w222 _] -> w205
              frame Disabled {
                n76 = call "Check if LineScan settings and LineScan image.vi"() -> ("LineScan Image?"=w222:bool, "LineScan settings?"=w223:bool)  [unwired: 10 in]
              }
              frame Enabled {
              }
            }
            n77 = case "Check for a calibration only is NOT inside a Line Scan" shown="Default" w204 {
              tunnel: w217 -> [_ w238]
              tunnel: w215 -> [_ w237]
              tunnel: [w226 w236] -> w214
              tunnel: [w225 w235] -> w213
              tunnel: w212 -> [w225 w234]
              tunnel: w211 -> [_ w233]
              tunnel: w210 -> [_ w232]
              tunnel: w209 -> [_ w231]
              tunnel: w208 -> [w226 _]
              tunnel: [TRUE _] -> w207
              tunnel: w206 -> [_ _]
              tunnel: w205 -> [_ _]
              frame "LineScan Settings" {
                n78 = disable-structure shown="Disabled" {
                  frame Disabled {
                    # "The Current Image has been generated from a Line Scan - Donot let the user mark points!"
                    n79 = property on="StimModuleStatus" class="Str"("Val(Sgnl)"="Cannot mark stim points on a Line Scan image!" ("Variable Name in")) -> ()  [unwired: 2 in, 2 out]
                  }
                  frame Enabled {
                  }
                }
              }
              frame Default {
                n80 = call "Check if Calibration valid for current parameters.vi"("System Information Cluster"=w238) -> ("Calibration Not Required?"=w228:bool, "Current Calibration Key"=w236:string, "Calibration Valid?"=w229:bool)  [unwired: 8 in]
                n81 = Or(x=w229, y=w228) -> (x .or. y?=w230:bool)
                n82 = case "Change UI behavior based on Calibration Availability" shown="True" w230 {
                  tunnel: w237 -> [_ w263]
                  tunnel: w236 -> [_ w260]
                  tunnel: [w239 w247] -> w235
                  tunnel: w234 -> [w239 _]
                  tunnel: w231 -> [_ w241]
                  tunnel: w233 -> [_ w251]
                  tunnel: w232 -> [_ w250]
                  frame False {
                    n83 = property on="StimModuleStatus" class="Str"("Val(Sgnl)"="Calibration unavailable for current scanner settings! Click on 'Calibrate' to start" ("Variable Name in")) -> ()  [unwired: 2 in, 2 out]
                  }
                  frame True {
                    # "update enabled stim points"
                    n84 = call "getPixelMapping.vi"("Key String IN"=w260) -> ("Rectangle"=w247:T14, "y.pixels"=w253:i32, "x.pixels"=w254:i32)  [unwired: 5 in, 3 out]
                    n85 = call "IMAQ GetImageSize"("Image"=w241) -> ("Y Resolution"=w256:i32, "X Resolution"=w257:i32)  [unwired: 3 in, 1 out]
                    n86 = property on="StimModuleStatus" class="Str"("Val(Sgnl)"="" ("Variable Name in")) -> ()  [unwired: 2 in, 2 out]
                    n87 = Equal?(x=w254, y=w257) -> (x = y?=w259:bool)
                    n88 = Equal?(x=w256, y=w253) -> (x = y?=w258:bool)
                    n89 = And(x=w259, y=w258) -> (x .and. y?=w255:bool)
                    n90 = call "Disable_stim_points_outside_stim_area.vi"("Current stim box"=w247, "Protocol Editor Ref IN"=w263) -> ("error out"=w261:errorcluster, "Protocol Editor Ref OUT"=w262:refnum<vi>)  [unwired: 8 in]
                    n91 = case shown="False" w255 {
                      tunnel: w241 -> [w271 w272]
                      tunnel: w254 -> [w267 _]
                      tunnel: w253 -> [w266 _]
                      tunnel: [w265 w272] -> w252
                      frame False {
                        n92 = call "Generate Static Image.vi"("Image Y Size"=w266, "Image X Size"=w267) -> ("error out"=w270:errorcluster, "Image 2"=w268:T1)  [unwired: 8 in]
                        n93 = call "IMAQ Copy"("error in (no error)"=w270, "Image Dst"=w271, "Image Src"=w268) -> ("error out"=w269:errorcluster, "Image Dst Out"=w265:T1)  [unwired: 3 in]
                        n94 = call "IMAQ Dispose"("Image"=w268, "error in (no error)"=w269) -> ()  [unwired: 4 in, 1 out]
                      }
                      frame True {
                      }
                    }
                    n95 = Close Reference(reference=w262, error in (no error)=w261) -> ()  [unwired: 1 out]
                    n96 = call "IMAQ Copy Overlay"("Image Dst"=w252, "Image Src"=w251) -> ("error out"=w242:errorcluster, "Image Dst Out"=w246:T1)  [unwired: 8 in]
                    n97 = call "IMAQ Clear Overlay"("error in (no error)"=w242, "Image"=w250) -> ("error out"=w243:errorcluster, "Image Out"=w248:T1)  [unwired: 8 in]
                    n98 = call "IMAQ Overlay Rectangle"("Color"=u32 6618880, "error in (no error)"=w243, "Rectangle"=w247, "Image"=w248) -> ("error out"=w244:errorcluster, "Image Out"=w245:T1)  [unwired: 6 in]
                    n99 = call "IMAQ Copy Overlay"("error in (no error)"=w244, "Image Dst"=w246, "Image Src"=w245) -> ()  [unwired: 7 in, 2 out]
                  }
                }
              }
            }
          }
          frame "stim in progress" {
            # "No Gated PMT support for Non-Hyperscope (Legacy) systems!"
            n100 = call-poly "GFGpolyGet.vi"("Variable Name in"="Hyperscope") -> ("Boolean Value OUT"=w273:bool)  [unwired: 9 in, 1 out]
            n101 = case shown="False" w273 {
              tunnel: w291 -> [_ w301]
              tunnel: [TRUE ("task done?") w300] -> w287
              tunnel: [_ w299] -> w282
              frame False {
              }
              frame True {
                n102 = call <vilib>:"DAQmx Is Task Done.vi"("task/channels in"=w301) -> ("task done?"=w300:bool, "error out"=w299:errorcluster)  [unwired: 12 in, 1 out]
              }
            }
            n103 = call <vilib>:"DAQmx Is Task Done.vi"("task/channels in"=w295) -> ("task done?"=w289:bool, "error out"=w284:errorcluster)  [unwired: 12 in, 1 out]
            n104 = call <vilib>:"DAQmx Is Task Done.vi"("task/channels in"=w292) -> ("task done?"=w288:bool, "error out"=w283:errorcluster)  [unwired: 12 in, 1 out]
            n105 = Merge Errors(w284, w283, w282) -> (w281:errorcluster)
            n106 = Compound Arithmetic op=AND(w289, w288, w287) -> (w290:bool)
            n107 = call <vilib>:"Clear Errors.vi"("error in (no error)"=w281) -> ()  [unwired: 6 in, 1 out]
            n108 = case shown="True" w290 {
              tunnel: [w305 -1] -> w280
              tunnel: w295 -> [w306 w319]
              tunnel: w292 -> [w307 w318]
              tunnel: [w307 refnum<k21> refnum ("task out")] -> w297
              tunnel: [w306 refnum<k21> refnum ("task out")] -> w296
              tunnel: w285 -> [w305 _]
              tunnel: w291 -> [w304 w313]
              tunnel: [w304 refnum<k21> refnum ("task out")] -> w294
              tunnel: [w303 w311] -> w293
              tunnel: w286 -> [w303 _]
              tunnel: w279 -> [w302 _]
              tunnel: [w302 _] -> w278
              tunnel: w275 -> [_ w308]
              frame False {
              }
              frame True {
                w315 = T12."Enabled" ("Disabled")
                # "Tasks complete; So clear tasks"
                n109 = call <vilib>:"DAQmx Clear Task.vi"("task in"=w313) -> ()  [unwired: 14 in, 1 out]
                n110 = call <vilib>:"DAQmx Clear Task.vi"("task in"=w318) -> ()  [unwired: 14 in, 1 out]
                n111 = call <vilib>:"DAQmx Clear Task.vi"("task in"=w319) -> ()  [unwired: 14 in, 1 out]
                n112 = property on="Uncage ONLY" class="Bool (strict)"("DisabledEnum"=w315) -> ()  [unwired: 2 in, 2 out]
                n113 = property on="Uncage and Image" class="Bool (strict)"("DisabledEnum"=w315) -> ()  [unwired: 2 in, 2 out]
                n114 = flat-sequence {
                  tunnel: [FALSE ("Value (Signaling)")] -> w311
                  frame #0 {
                    n115 = call "reset AO_galvo_stim.vi"() -> ()  [unwired: 11 in, 1 out]
                  }
                  frame #1 {
                    n116 = property on="Uncage and Image" class="Bool (strict)"("Value"=FALSE ("Uncage and Image")) -> ()  [unwired: 2 in, 2 out]
                    n117 = property on="Uncage ONLY" class="Bool (strict)"("Value"=FALSE ("Uncage ONLY")) -> ()  [unwired: 2 in, 2 out]
                  }
                  frame #2 {
                  }
                }
                n118 = case "If same Stim and Im Path; reset Pockels voltage to the last scan voltage set by the user from SciScan GUI" shown="True" w308 {
                  frame False {
                  }
                  frame True {
                    (unwired) 0.0 ("Numeric")
                    w322 = "Laser.Power" ("Variable Name in")
                    n119 = call "GFGnumericGet.vi"("Variable Name in"=w322) -> ("Numeric"=w321:dbl)  [unwired: 8 in, 2 out]
                    n120 = call "GFG_core.vi"("Variable Name in"=w322, "Variant in"=w321, "Action"=enum16{"Init", "Set", "Get", "Clear"}."Set") -> ()  [unwired: 10 in, 7 out]
                  }
                }
                n121 = property on="Uncaging Shutter" class="Bool (strict)"("Val(Sgnl)"=FALSE ("Value (Signaling)")) -> ()  [unwired: 2 in, 2 out]
                n122 = call-poly "GFGpolyGet.vi"("Variable Name in"="Hyperscope.type") -> ("String"=w310:string)  [unwired: 9 in, 1 out]
                n123 = case "Special Case for RGG where Pockels sits on PCI 6110" shown="\"RGG\"" w310 {
                  frame "False", Default {
                  }
                  frame "RGG" {
                    n124 = call "Timebase and Trigger Routing.vi"("Signal Router Action"=Timebase_and_Trigger_Routing."Disconnect all", "System Type"="Stimulation Only (RGG Case)" ("Variable Name in")) -> ()  [unwired: 9 in, 1 out]
                  }
                }
              }
            }
          }
        }
      }
      event "Image1": Mouse Down {
        w345 = u32 1  # Point tool
        w342 = u16 1  # Left mouse button
        # "valid calib key \nor calib not required?"
        n125 = event-data() -> ("Button"=w352:u16)  [unwired: 1 in]
        n126 = property class="ImageControl"(reference=w334) -> ("Current ROI Tool"=w341:u32)  [unwired: 1 in, 2 out]
        n127 = property class="ImageControl" props=["Current ROI Tool"](reference=w334) -> ()  [unwired: 1 in, 3 out]
        n128 = property on="Image1" class="ImageControl"() -> ("Last Mouse Position"=w348:cluster{"X":i32, "Y":i32})  [unwired: 2 in, 2 out]
        n129 = Equal?(x=w342, y=w352) -> (x = y?=w344:bool)
        n130 = Empty String/Path?(string/path=w338) -> (empty?=w339:bool)
        n131 = Equal?(x=w345, y=w341) -> (x = y?=w343:bool)
        n132 = feedback #1() -> (w349:cluster{"X":i32, "Y":i32})  [unwired: 1 in]
        n133 = feedback-in #1(w348) -> ()
        n134 = Not(x=w339) -> (.not. x?=w331:bool)
        n135 = Or(x=w331, y=w330) -> (x .or. y?=w332:bool)
        n136 = Not Equal?(x=w349, y=w348) -> (x != y?=w347:bool)
        n137 = Compound Arithmetic op=AND(w346, w343, w344, w347, w332) -> (w351:bool)
        n138 = case shown="True" w351 {
          tunnel: [w367 w382] -> w365
          tunnel: w364 -> [w367 w381]
          tunnel: w360 -> [_ w371]
          tunnel: w359 -> [_ w380]
          tunnel: w358 -> [_ w379]
          tunnel: w357 -> [_ w378]
          tunnel: w354 -> [w366 w374]
          tunnel: [w366 w376] -> w353
          tunnel: w350 -> [_ w377]
          tunnel: w348 -> [_ w373]
          tunnel: w338 -> [_ w372]
          tunnel: w329 -> [_ w368]
          frame False {
          }
          frame True {
            n139 = call "Check if same stim and Imaging Path.vi"("System Information Cluster"=w368) -> ("Boolean"=w369:bool)  [unwired: 10 in]
            n140 = case shown="False" w369 {
              tunnel: [w385 TRUE] -> w375
              tunnel: w373 -> [w383 w395]
              tunnel: w372 -> [w384 _]
              tunnel: [w383 w395] -> w370
              frame False {
                # "Check, if the selected stimulation point is in the boundary of the stimulatable area"
                n141 = call "getPixelMapping.vi"("Key String IN"=w384) -> ("Rectangle"=w386:T14)  [unwired: 5 in, 5 out]
                n142 = Unbundle By Name(w386) -> ("Left"=w387:i32, "Top"=w391:i32, "Right"=w389:i32, "Bottom"=w392:i32)
                n143 = Unbundle By Name(w383) -> ("X"=w388:i32, "Y"=w390:i32)
                n144 = In Range and Coerce(upper limit=w389, x=w388, lower limit=w387) -> (In Range?=w393:bool)  [unwired: 1 out]
                n145 = In Range and Coerce(upper limit=w392, x=w390, lower limit=w391) -> (In Range?=w394:bool)  [unwired: 1 out]
                n146 = And(x=w393, y=w394) -> (x .and. y?=w385:bool)
              }
              frame True {
                # "Stim path = Imaging path - no bounding box required!"
              }
            }
            n147 = case shown="True" w375 {
              tunnel: [w398 w461] -> w382
              tunnel: w381 -> [w398 _]
              tunnel: w380 -> [_ w426]
              tunnel: w379 -> [_ w419]
              tunnel: w371 -> [_ w417]
              tunnel: w378 -> [_ w412]
              tunnel: w377 -> [_ w411]
              tunnel: [w397 w410] -> w376
              tunnel: w370 -> [_ w409]
              tunnel: w374 -> [w397 _]
              frame False {
                n148 = One Button Dialog(message="The point you have selected is outside the area you can stimulate.") -> ()  [unwired: 1 in, 1 out]
              }
              frame True {
                w408 = "%^.0p" ("format string")
                # "New Code - FAST update of ROI"
                n149 = property on="Protocol Editor" class="MCListbox (strict)"() -> ("ItemNames"=w458:string[][])  [unwired: 2 in, 2 out]
                n150 = case shown="False" w411 {
                  tunnel: [w463 FALSE ("Waveform changed!")] -> w410
                  frame False {
                    w463 = TRUE  # Waveform changed!
                  }
                  frame True {
                    n151 = property on="Update waveform and Timing" class="Bool (strict)"("Val(Sgnl)"=TRUE ("Value (Signaling)")) -> ()  [unwired: 2 in, 2 out]
                  }
                }
                n152 = global read "save ROI.vi" "Save Coordinates"() -> (w443:T10)
                n153 = Index Array(array=w458, index (col)=0 ("index (row)")) -> (element=w455:string[])  [unwired: 1 in]
                n154 = Unbundle By Name(w409) -> ("X"=w452:i32, "Y"=w451:i32)
                n155 = Unbundle By Name(w409) -> ("Y"=w422:i32)
                n156 = for {
                  tunnel: w455 -> [w468] mode=indexing
                  tunnel: [w466] -> w457 mode=indexing
                  n157 = Scan From String(format string="%d", input string=w468) -> (output 1=w466:i32)  [unwired: 3 in, 3 out]
                }
                n158 = Add(x=w422, y=w412) -> (x+y=w421:i32)
                n159 = Bundle By Name(cluster=w409, "Y"=w421) -> (w420:cluster{"X":i32, "Y":i32})
                n160 = Array Max & Min(array=w457) -> (max value=w456:i32)  [unwired: 3 out]
                n161 = Increment(x=w456) -> (x+1=w462:i32)
                n162 = Number To Decimal String(number=w462) -> (decimal integer string=w442:string)  [unwired: 1 in]
                n163 = Number To Decimal String(number=w452) -> (decimal integer string=w449:string)  [unwired: 1 in]
                n164 = Number To Decimal String(number=w451) -> (decimal integer string=w448:string)  [unwired: 1 in]
                n165 = call "IMAQ Convert Point to ROI"("Point"=w409) -> ("ROI Descriptor"=w415:T30)  [unwired: 8 in, 1 out]
                n166 = Concatenate Strings(w442, "[" ("string"), w449, "," ("string"), w448, "]" ("string")) -> (w416:string)
                n167 = Search/Split String(string=w416, search string/char (-)="[" ("regular expression")) -> (substring before match=w413:string)  [unwired: 1 in, 2 out]
                n168 = call "IMAQ Overlay ROI"("Colors (Green)"=u32[] [65280], "Group"=w413, "Point Symbol"=w419, "ROI Descriptor"=w415, "Image"=w426) -> ("Image Out"=w423:T1)  [unwired: 5 in, 1 out]
                n169 = Bundle By Name(cluster=T16 {"ROI name"="", "pixel coordinates"={"x"=0, "y"=0}} ("notebook"), "ROI name"=w416, "pixel coordinates.x"=w452, "pixel coordinates.y"=w451) -> (w445:T16)
                n170 = call "IMAQ Overlay Text"("Group"=w413, "Text Color (black)"=u32 16711680, "String"=w413, "Origin"=w420, "Image"=w423) -> ("Image Out"=w414:T1)  [unwired: 5 in, 1 out]
                n171 = Build Array (concatenate)(w443, w445) -> (w444:T10)
                n172 = call "IMAQ Copy Overlay"("Image Dst"=w417, "Image Src"=w414) -> ()  [unwired: 8 in, 2 out]
                n173 = global write "save ROI.vi" "Save Coordinates"(w444) -> ()
                n174 = property on="Protocol Editor" class="MCListbox (strict)"() -> ("ItemNames"=w405:string[][], "ItemSyms"=w401:i32[])  [unwired: 2 in, 2 out]
                n175 = Index Array(array=w405, index (col)=0 ("disabled index (col)")) -> (element=w403:string[])  [unwired: 1 in]
                n176 = Build Array (concatenate)(w401, 38) -> (w446:i32[])
                n177 = Build Array (concatenate)(w403, w416) -> (w402:string[])
                n178 = Array Subset(array=w405, index (row)=0 ("index"), index (col)=1 ("index")) -> (w460:string[][])  [unwired: 2 in]
                n179 = call "save coor order.vi"("Save Coordinates"=w444, "Stm ID"=w402) -> ("New ROI"=w454:string[])  [unwired: 9 in]
                n180 = Format Into String(format string=w408, "Stim duration (s)") -> (resulting string=w435:string)  [unwired: 2 in, 1 out]
                n181 = Format Into String(format string=w408, "Stim interval (s)") -> (resulting string=w431:string)  [unwired: 2 in, 1 out]
                n182 = Number To Decimal String(number="Spot repetitions") -> (decimal integer string=w430:string)  [unwired: 1 in]
                n183 = Format Into String(format string=w408, "Stim Power (%)") -> (resulting string=w429:string)  [unwired: 2 in, 1 out]
                n184 = Format Into String(format string=w408, "Pre-stim settling time (s)") -> (resulting string=w427:string)  [unwired: 2 in, 1 out]
                n185 = Build Array(w435, w431, w430, w429, w427) -> (w437:string[])
                n186 = Build Array (concatenate)(w460, w437) -> (w461:string[][])
                n187 = Transpose 2D Array(2D array=w461) -> (transposed array=w439:string[][])
                n188 = Build Array (concatenate)(w454, w439) -> (w440:string[][])
                n189 = Transpose 2D Array(2D array=w440) -> (transposed array=w438:string[][])
                n190 = property on="Protocol Editor" class="MCListbox (strict)"("ItemNames"=w438, "ItemSyms"=w446) -> ()  [unwired: 2 in, 2 out]
              }
            }
          }
        }
      }
      event "Image1": Mouse Leave {
        n191 = event-data() -> ()  [unwired: 1 in, 1 out]
      }
      event "Image1": Mouse Enter {
        n192 = event-data() -> ()  [unwired: 1 in, 1 out]
      }
      event "reset zoom_Photo-Stim_UI": Value Change {
        n193 = event-data() -> ()  [unwired: 1 in, 1 out]
        n194 = property class="ImageControl"(reference=w505, "Zoom to Fit Mode"=TRUE) -> ()  [unwired: 1 in, 2 out]
      }
      event User Event {
        n195 = event-data() -> ("Variable Name"=w539:string, "Variant"=w538:variant, "Source VI"=w528:string)  [unwired: 1 in]
        n196 = case shown="\"CurrentImageType\"" w539 {
          selector: w539 -> [_ _ w618 _ _ _ _ _ _ _]
          tunnel: w538 -> [_ w548 w619 _ _ _ _ w791 w810 _]
          tunnel: w537 -> [_ w559 _ _ w647 _ _ _ _ _]
          tunnel: w535 -> [_ w558 _ _ w657 _ _ _ _ _]
          tunnel: [_ _ _ _ _ _ _ _ _ TRUE] -> w534
          tunnel: w533 -> [_ w557 _ _ _ _ _ _ _ _]
          tunnel: w532 -> [_ w556 _ _ w650 _ _ _ _ _]
          tunnel: w528 -> [_ _ _ _ w665 w770 _ _ _ _]
          tunnel: w527 -> [_ _ _ _ w666 _ _ _ _ _]
          tunnel: w526 -> [_ w555 _ w631 w662 _ _ _ _ _]
          tunnel: w524 -> [_ _ _ _ _ _ _ _ _ _]
          tunnel: w523 -> [w545 w549 w623 w632 w664 w765 w781 w792 w808 w819]
          tunnel: [w545 w549 w623 w632 w664 w765 w780 w792 w808 w819] -> w522
          tunnel: w521 -> [w543 w553 w621 w625 w645 w763 w782 w789 w806 w817]
          tunnel: w520 -> [_ _ _ w630 w663 _ _ _ _ _]
          tunnel: w517 -> [w544 w552 w622 w626 w646 w764 w779 _ w807 w818]
          tunnel: [w544 w552 w622 w626 w646 w764 w779 w790 w807 w818] -> w516
          tunnel: [w543 w553 w621 w625 w645 w763 w778 w789 w806 w817] -> w515
          tunnel: w514 -> [w542 w551 w620 w624 w642 w762 w777 w788 w805 w816]
          tunnel: [w542 w550 w620 w624 w642 w762 w777 w788 w805 w816] -> w513
          tunnel: [_ _ w618 _ _ _ _ _ _ _] -> _
          tunnel: [_ _ w619 _ _ _ _ _ _ _] -> _
          frame "False", Default {
          }
          frame "CurrentImageType" {
            n197 = disable-structure shown="Enabled" {
              disable-tunnel: w557 -> [w565 _]
              disable-tunnel: [w560 TRUE] -> w554
              frame Enabled {
                # "Refresh time elapsed?"
                n198 = Get Date/Time In Seconds() -> (seconds since 1Jan1904=w564:timestamp)
                n199 = feedback #2() -> (w562:timestamp)  [unwired: 1 in]
                n200 = Subtract(x=w564, y=w562) -> (x-y=w566:dbl)
                n201 = Greater?(x=w566, y=w565) -> (0:w561:bool)
                n202 = case shown="False" w561 {
                  selector: w561 -> [w567 w569]
                  tunnel: w564 -> [_ w570]
                  tunnel: [w568 w570] -> w563
                  tunnel: w562 -> [w568 _]
                  tunnel: [w567 w569] -> w560
                  frame False {
                  }
                  frame True {
                  }
                }
                n203 = feedback-in #2(w563) -> ()
              }
              frame Disabled {
                # "Refresh Every frame!"
              }
            }
            n204 = Variant To Data(type=Image_Types."Frame Scan" ("Image Types"), Variant=w548) -> (data=w546:T17)  [unwired: 1 in, 1 out]
            n205 = case shown="\"Frame Scan\", \"ROI\"" w546 {
              tunnel: w559 -> [_ w580 _]
              tunnel: w558 -> [_ w579 _]
              tunnel: w556 -> [_ w578 _]
              tunnel: w555 -> [_ w577 _]
              tunnel: w554 -> [_ w576 _]
              tunnel: w552 -> [_ w575 _]
              tunnel: w551 -> [w572 w574 _]
              tunnel: [w572 w573 LineScan_Image_Status."LineScan  image" ("t")] -> w550
              frame Default {
                # "Update the Image only if it is a Frame Scan"
              }
              frame "Frame Scan", "ROI" {
                n206 = case shown="True" w576 {
                  tunnel: w580 -> [_ w588]
                  tunnel: w579 -> [_ w595]
                  tunnel: w578 -> [_ w586]
                  tunnel: w577 -> [_ w585]
                  tunnel: w575 -> [_ _]
                  tunnel: w574 -> [w581 w584]
                  tunnel: [w581 w583] -> w573
                  frame False {
                  }
                  frame True {
                    w593 = refnum<vi> refnum  # Generic
                    # "Is Current Image a LineScan Image?"
                    n207 = To More Generic Class(target class=w593, reference=w595) -> (generic class reference=w594:refnum<vi>)
                    n208 = call "getSciScan image reference.vi"("Image Refnum (Generic)"=w594) -> ("Current Image"=w587:T1, "Channel type"=w582:string)  [unwired: 6 in, 3 out]
                    n209 = case "If LineScan settings; new image IN THE LINESCAN image tab is a lineScan image which is invalid for point selection!" shown="\"channel arb line scan\"" w582 {
                      tunnel: w584 -> [_ w616]
                      tunnel: [LineScan_Image_Status."not a LineScan image" ("t") w616] -> w583
                      frame "channel arb line scan" {
                      }
                      frame Default {
                      }
                    }
                    n210 = Equal?(x=T1 refnum, y=w587) -> (x = y?=w591:bool)
                    n211 = call "IMAQ GetImageSize"("Image"=w588) -> ("Y Resolution"=w589:i32, "X Resolution"=w590:i32)  [unwired: 3 in, 1 out]
                    n212 = case shown="False" w591 {
                      tunnel: w590 -> [w606 _]
                      tunnel: w589 -> [w605 _]
                      tunnel: w588 -> [w602 w612]
                      tunnel: w587 -> [_ w611]
                      tunnel: w586 -> [w600 w610]
                      tunnel: w585 -> [w601 w609]
                      frame True {
                        n213 = call "Generate Static Image.vi"("Image Y Size"=w605, "Image X Size"=w606) -> ("Image 2"=w598:T1)  [unwired: 8 in, 1 out]
                        n214 = call "IMAQ Copy"("Image Dst"=w602, "Image Src"=w598) -> ("error out"=w604:errorcluster, "Image Dst Out"=w603:T1)  [unwired: 4 in]
                        n215 = call "IMAQ Copy Overlay"("error in (no error)"=w604, "Image Dst"=w603, "Image Src"=w600) -> ("error out"=w597:errorcluster, "Image Dst Out"=w596:T1)  [unwired: 7 in]
                        n216 = call "IMAQ Copy Overlay"("error in (no error)"=w597, "Image Dst"=w596, "Image Src"=w601) -> ("error out"=w599:errorcluster)  [unwired: 7 in, 1 out]
                        n217 = call "IMAQ Dispose"("Image"=w598, "error in (no error)"=w599) -> ()  [unwired: 4 in, 1 out]
                      }
                      frame False {
                        n218 = call "IMAQ Copy"("Image Dst"=w612, "Image Src"=w611) -> ("error out"=w614:errorcluster, "Image Dst Out"=w613:T1)  [unwired: 4 in]
                        n219 = call "IMAQ Copy Overlay"("error in (no error)"=w614, "Image Dst"=w613, "Image Src"=w610) -> ("error out"=w608:errorcluster, "Image Dst Out"=w607:T1)  [unwired: 7 in]
                        n220 = call "IMAQ Copy Overlay"("error in (no error)"=w608, "Image Dst"=w607, "Image Src"=w609) -> ()  [unwired: 7 in, 2 out]
                      }
                    }
                  }
                }
              }
              frame "Line Scan" {
              }
            }
          }
          frame "channel.no" {
          }
          frame "FOCUS", "Record" {
            # "Redraw bounding rectangle"
            # "clear bounding rectangle"
            n221 = call "IMAQ Clear Overlay"("Image"=w631) -> ("Image Out"=w627:T1)  [unwired: 9 in, 1 out]
            n222 = call "getPixelMapping.vi"("Key String IN"=w630) -> ("Rectangle"=w629:T14, "Calibration Available?"=w628:bool)  [unwired: 5 in, 4 out]
            n223 = case shown="True" w628 {
              tunnel: w627 -> [w633 w636]
              tunnel: w629 -> [_ w635]
              tunnel: [w633 w634] -> _
              frame False {
              }
              frame True {
                n224 = call "IMAQ Overlay Rectangle"("Color"=u32 6618880, "Rectangle"=w635, "Image"=w636) -> ("Image Out"=w634:T1)  [unwired: 7 in, 1 out]
              }
            }
          }
          frame "MAIN.Image.panels.", "MAIN.Image.panels.reso.", "ROI.channel", "channel.arb.line.scan" {
            w658 = refnum<vi> refnum  # Generic
            n225 = To More Generic Class(target class=w658, reference=w657) -> (generic class reference=w656:refnum<vi>)
            n226 = call "getSciScan image reference.vi"("Image Refnum (Generic)"=w656) -> ("Channel Number"=w648:u32, "Current Image"=w652:T1, "Channel type"=w643:string)  [unwired: 6 in, 2 out]
            n227 = Equal?(x=T1 refnum, y=w652) -> (x = y?=w649:bool)
            n228 = Equal?(x=w643, y="channel arb line scan" ("Channel type")) -> (x = y?=w639:bool)
            n229 = call "IMAQ GetImageSize"("Image"=w647) -> ("Y Resolution"=w653:i32, "X Resolution"=w654:i32)  [unwired: 3 in, 1 out]
            n230 = case shown="Default" w643 {
              tunnel: w666 -> [w711 w722 w731]
              tunnel: w665 -> [w710 _ _]
              tunnel: w648 -> [w701 _ w728]
              frame "regular channel" {
                n231 = control-ref of="This VI"() -> (w709:refnum<vi>)
                n232 = property class="VI"(reference=w709) -> (reference out=w706:refnum<vi>, error out=w707:errorcluster, "Name"=w708:string)  [unwired: 1 in]
                n233 = Decrement(x=w701) -> (x-1=w702:u32)
                n234 = Close Reference(reference=w706, error in (no error)=w707) -> ()  [unwired: 1 out]
                n235 = Not Equal?(x=w708, y=w710) -> (x != y?=w705:bool)
                n236 = case "Trigger a Tab Change if not initiated by this VI (else infinite loop!)" shown="True" w705 {
                  tunnel: w711 -> [w712 w716]
                  tunnel: [w712 w715] -> w704
                  tunnel: [_ w714] -> w703
                  tunnel: w702 -> [_ w713]
                  frame False {
                  }
                  frame True {
                    n237 = property class="TabCtl (strict)"(reference=w716, "Val(Sgnl)"=w713) -> (reference out=w715:refnum<vi>, error out=w714:errorcluster)  [unwired: 1 in]
                  }
                }
                n238 = Close Reference(reference=w704, error in (no error)=w703) -> ()  [unwired: 1 out]
              }
              frame Default {
                w717 = 5460819  # Grey
                n239 = property class="TabCtl (strict)"(reference=w722) -> (reference out=w720:refnum<vi>, "Value"=w719:T2)  [unwired: 1 in, 1 out]
                n240 = Build Array(w719) -> (w718:T31)
                n241 = Build Array(w717) -> (w721:i32[])
                n242 = for "Uncolour old tab and color new tab" {
                  tunnel: w720 -> [w727]
                  tunnel: w718 -> [w725] mode=indexing
                  tunnel: w721 -> [w726] mode=indexing
                  n243 = Build Array(w725) -> (w724:T31)
                  n244 = call "Change tab page colour.vi"("Action"=T8."Change specific tabs", "New Colour"=w726, "Page Indices"=w724, "TabControl in"=w727) -> ()  [unwired: 7 in, 1 out]
                }
              }
              frame "ROI channel", "channel arb line scan" {
                n245 = Decrement(x=w728) -> (x-1=w730:u32)
                n246 = Equal To 0?(x=w728) -> (x = 0?=w729:bool)
                n247 = case shown="False" w729 {
                  tunnel: w731 -> [w736 w746]
                  tunnel: w730 -> [w732 _]
                  frame False {
                    w737 = 5460819  # Grey
                    n248 = property class="TabCtl (strict)"(reference=w736) -> (reference out=w734:refnum<vi>, "Value"=w739:T2)  [unwired: 1 in, 1 out]
                    n249 = Build Array(w739, w732) -> (w738:u32[])
                    n250 = Build Array(w737, u32 0) -> (w740:u32[])
                    n251 = property class="TabCtl (strict)"(reference=w734, "Value"=w732) -> (reference out=w733:refnum<vi>)  [unwired: 1 in, 1 out]
                    n252 = for "Uncolour old tab and color new tab" {
                      tunnel: w733 -> [w745]
                      tunnel: w738 -> [w743] mode=indexing
                      tunnel: w740 -> [w744] mode=indexing
                      n253 = Build Array(w743) -> (w742:u32[])
                      n254 = call "Change tab page colour.vi"("Action"=T8."Change specific tabs", "New Colour"=w744, "Page Indices"=w742, "TabControl in"=w745) -> ()  [unwired: 7 in, 1 out]
                    }
                  }
                  frame True {
                    w747 = 5460819  # Grey
                    n255 = property class="TabCtl (strict)"(reference=w746) -> (reference out=w750:refnum<vi>, "Value"=w749:T2)  [unwired: 1 in, 1 out]
                    n256 = Build Array(w749) -> (w748:T31)
                    n257 = Build Array(w747) -> (w751:i32[])
                    n258 = for "Uncolour old tab and color new tab" {
                      tunnel: w750 -> [w756]
                      tunnel: w748 -> [w754] mode=indexing
                      tunnel: w751 -> [w755] mode=indexing
                      n259 = Build Array(w754) -> (w753:T31)
                      n260 = call "Change tab page colour.vi"("Action"=T8."Change specific tabs", "New Colour"=w755, "Page Indices"=w753, "TabControl in"=w756) -> ()  [unwired: 7 in, 1 out]
                    }
                  }
                }
              }
            }
            n261 = Equal?(x=LineScan_Image_Status."LineScan  image", y=w642) -> (x = y?=w640:bool)
            n262 = And(x=w639, y=w640) -> (x .and. y?=w638:bool)
            n263 = call "IMAQ Clear Overlay"("Image"=w662) -> ("Image Out"=w659:T1)  [unwired: 9 in, 1 out]
            n264 = call "getPixelMapping.vi"("Key String IN"=w663) -> ("Rectangle"=w661:T14, "Calibration Available?"=w660:bool)  [unwired: 5 in, 4 out]
            n265 = case shown="True" w660 {
              tunnel: w659 -> [w757 w760]
              tunnel: w661 -> [_ w759]
              tunnel: [w757 w758] -> w651
              frame False {
              }
              frame True {
                n266 = call "IMAQ Overlay Rectangle"("Color"=u32 6618880, "Rectangle"=w759, "Image"=w760) -> ("Image Out"=w758:T1)  [unwired: 7 in, 1 out]
              }
            }
            n267 = case "Donot Pull in a LineScan Image!!" shown="False" w638 {
              tunnel: w654 -> [w673 _]
              tunnel: w653 -> [w672 _]
              tunnel: w652 -> [w671 _]
              tunnel: w651 -> [w670 _]
              tunnel: w650 -> [w669 _]
              tunnel: w649 -> [w668 _]
              tunnel: w647 -> [w667 _]
              frame False {
                n268 = case shown="False" w668 {
                  tunnel: w673 -> [w678 _]
                  tunnel: w672 -> [w677 _]
                  tunnel: w667 -> [w681 w698]
                  tunnel: w671 -> [_ w697]
                  tunnel: w670 -> [w679 w696]
                  tunnel: w669 -> [w680 w695]
                  frame True {
                    n269 = Greater Than 0?(x=w678) -> (x > 0?=w675:bool)
                    n270 = Greater Than 0?(x=w677) -> (x > 0?=w674:bool)
                    n271 = And(x=w675, y=w674) -> (x .and. y?=w676:bool)
                    n272 = case shown="True" w676 {
                      tunnel: w678 -> [_ w692]
                      tunnel: w677 -> [_ w691]
                      tunnel: w681 -> [_ w688]
                      tunnel: w680 -> [_ w687]
                      tunnel: w679 -> [_ w686]
                      frame False {
                      }
                      frame True {
                        n273 = call "Generate Static Image.vi"("Image Y Size"=w691, "Image X Size"=w692) -> ("Image 2"=w684:T1)  [unwired: 8 in, 1 out]
                        n274 = call "IMAQ Copy"("Image Dst"=w688, "Image Src"=w684) -> ("error out"=w690:errorcluster, "Image Dst Out"=w689:T1)  [unwired: 4 in]
                        n275 = call "IMAQ Copy Overlay"("error in (no error)"=w690, "Image Dst"=w689, "Image Src"=w686) -> ("error out"=w683:errorcluster, "Image Dst Out"=w682:T1)  [unwired: 7 in]
                        n276 = call "IMAQ Copy Overlay"("error in (no error)"=w683, "Image Dst"=w682, "Image Src"=w687) -> ("error out"=w685:errorcluster)  [unwired: 7 in, 1 out]
                        n277 = call "IMAQ Dispose"("Image"=w684, "error in (no error)"=w685) -> ()  [unwired: 4 in, 1 out]
                      }
                    }
                  }
                  frame False {
                    n278 = call "IMAQ Copy"("Image Dst"=w698, "Image Src"=w697) -> ("error out"=w700:errorcluster, "Image Dst Out"=w699:T1)  [unwired: 4 in]
                    n279 = call "IMAQ Copy Overlay"("error in (no error)"=w700, "Image Dst"=w699, "Image Src"=w696) -> ("error out"=w694:errorcluster, "Image Dst Out"=w693:T1)  [unwired: 7 in]
                    n280 = call "IMAQ Copy Overlay"("error in (no error)"=w694, "Image Dst"=w693, "Image Src"=w695) -> ()  [unwired: 7 in, 2 out]
                  }
                }
              }
              frame True {
              }
            }
          }
          frame "Cancel" {
            # "Received a 'Cancel' Command from SciScan.\nIf any Photostim tasks are running; Hit a Cancel to Stop it and carry out unrouting and other relevant cleanup"
            n281 = control-ref of="This VI"() -> (w771:refnum<vi>)
            n282 = property class="VI"(reference=w771) -> ("Name"=w769:string)  [unwired: 1 in, 2 out]
            n283 = Not Equal?(x=w770, y=w769) -> (x != y?=w767:bool)
            n284 = property on="Uncage and Image" class="Bool (strict)"() -> ("Value"=w773:bool)  [unwired: 2 in, 2 out]
            n285 = property on="Uncage ONLY" class="Bool (strict)"() -> ("Value"=w772:bool)  [unwired: 2 in, 2 out]
            n286 = Or(x=w772, y=w773) -> (x .or. y?=w768:bool)
            n287 = And(x=w768, y=w767) -> (x .and. y?=w766:bool)
            n288 = case shown="True" w766 {
              tunnel: w772 -> [_ w774]
              frame False {
              }
              frame True {
                n289 = case shown="True" w774 {
                  frame False {
                    n290 = property on="Uncage and Image" class="Bool (strict)"("Val(Sgnl)"=FALSE ("Uncage and Image")) -> ()  [unwired: 2 in, 2 out]
                  }
                  frame True {
                    n291 = property on="Uncage ONLY" class="Bool (strict)"("Val(Sgnl)"=FALSE ("Uncage ONLY")) -> ()  [unwired: 2 in, 2 out]
                  }
                }
              }
            }
          }
          frame "Flag_CalibrationChanged", "Start.Delay", "fill.fraction", "nomin.x.pixels", "speed.mode", "x.bidirectional", "x.invert.image", "x.volt.offset", "x.voltage", "y.bidirectional", "y.invert.image", "y.pixels", "y.volt.offset", "y.voltage" {
            n292 = case shown="Default" w782 {
              selector: w782 -> [w783 w787]
              tunnel: w781 -> [_ w786]
              tunnel: [w784 w787] -> w778
              tunnel: [50 w786] -> w780
              tunnel: [w783 _] -> _
              frame Default {
                w784 = "calibration change"  # Polling Type
                # "GFG variables indicating a change of calibration.\ncheck calibration status!\n\nHandler in Timeout case"
              }
              frame "stim in progress" {
                # "A stim is in progress - ignore the calibration check!"
              }
            }
          }
          frame "scan.mode.main.settings" {
            # "If LineScan tab selected by user - update flag to 'LineScanSettings'"
            # "Check if on the LineScan Tab"
            n293 = disable-structure shown="Disabled" {
              disable-tunnel: w791 -> [w799 _]
              disable-tunnel: [w793 w804] -> w790
              frame Enabled {
                w803 = scan_mode_main_settings_tab."2D frame"  # scan mode main settings
                n294 = call "GFG_core.vi"("Variable Name in"="scan.mode.main.settings", "Variant in"=w799, "Action"=enum16{"Init", "Set", "Get", "Clear"}."Get") -> ("Variant Out"=w802:variant)  [unwired: 10 in, 6 out]
                n295 = Variant To Data(type=w803, Variant=w802) -> (data=w797:T18)  [unwired: 1 in, 1 out]
                n296 = Equal?(x=scan_mode_main_settings_tab."2D line scan", y=w797) -> (x = y?=w796:bool)
                n297 = Select(t=LineScan_settings_Status."LineScan Settings" ("LineScan Status"), s=w796, f=LineScan_settings_Status."not Linescan Settings" ("LineScan Status")) -> (s? t:f=w793:T5)
              }
              frame Disabled {
              }
            }
          }
          frame "shutter" {
            n298 = Variant To Data(type=FALSE, Variant=w810) -> (data=w809:bool)  [unwired: 1 in, 1 out]
            n299 = call-poly "GFGpolyGet.vi"("Variable Name in"="scanner.type") -> ("String"=w812:string)  [unwired: 9 in, 1 out]
            n300 = case shown="\"Imaging Path Galvo\", \"Imaging Path Reso\"" w812 {
              tunnel: w809 -> [w814 w815 _]
              frame "Imaging Path Galvo", "Imaging Path Reso" {
                n301 = property on="Imaging Shutter" class="Bool (strict)"("Value"=w814) -> ()  [unwired: 2 in, 2 out]
              }
              frame "Stimulation Path Galvo" {
                n302 = property on="Uncaging Shutter" class="Bool (strict)"("Value"=w815) -> ()  [unwired: 2 in, 2 out]
              }
              frame Default {
              }
            }
          }
          frame "QUIT" {
          }
        }
      }
      event "Uncaging Shutter": Value Change {
        n303 = event-data() -> ("NewVal"=w830:bool)  [unwired: 1 in]
        n304 = call-poly "GFGpolyGet.vi"("Variable Name in"="scanner.type") -> ("String"=w831:string)  [unwired: 9 in, 1 out]
        n305 = case shown="\"Stimulation Path Galvo\"" w831 {
          tunnel: w830 -> [_ w840]
          frame Default {
          }
          frame "Stimulation Path Galvo" {
            # "Update Shutter in  the Main SciScan UI"
            n306 = call "GFG_core.vi"("Variable Name in"="shutter", "Variant in"=w840, "Action"=enum16{"Init", "Set", "Get", "Clear"}."Set") -> ()  [unwired: 10 in, 7 out]
          }
        }
        n307 = call "GFG_core.vi"("Variable Name in"="Uncaging.Shutter", "Variant in"=w830, "Action"=enum16{"Init", "Set", "Get", "Clear"}."Set") -> ()  [unwired: 10 in, 7 out]
      }
      event "Channel Selector": Value Change {
        w854 = 5460819  # Grey
        n308 = event-data() -> ("OldVal"=w850:T2, "NewVal"=w849:T2)  [unwired: 1 in]
        n309 = Build Array(w850, w849) -> (w856:T31)
        n310 = call "Query if Galvo or Reso.vi"() -> ("System Type"=w855:enum16{"Galvo", "Reso"})  [unwired: 10 in, 1 out]
        n311 = Build Array(w854, u32 0 ("New Colour")) -> (w852:u32[])
        n312 = case "Update Channel Selection in SciScan" shown="\"Galvo\"" w855 {
          tunnel: w849 -> [w872 w878]
          frame "Reso" {
            w873 = MAIN_Image_panel_reso_tab_Control_type_def."Channel 1"  # MAIN Image panels reso
            n313 = Type Cast(type=w873, x=w872) -> (*(type *) &x=w871:T32)
            n314 = call "GFG_core.vi"("Variable Name in"="MAIN Image panels reso ", "Variant in"=w871, "Action"=enum16{"Init", "Set", "Get", "Clear"}."Set") -> ()  [unwired: 10 in, 7 out]
          }
          frame "Galvo" {
            w875 = MAIN_Image_panel_tab_Control_type_def."Channel 1"  # MAIN Image panels
            n315 = Type Cast(type=w875, x=w878) -> (*(type *) &x=w877:T33)
            n316 = call "GFG_core.vi"("Variable Name in"="MAIN Image panels ", "Variant in"=w877, "Action"=enum16{"Init", "Set", "Get", "Clear"}."Set") -> ()  [unwired: 10 in, 7 out]
          }
        }
        n317 = for "Uncolour old tab and color new tab" {
          tunnel: w851 -> [w869]
          tunnel: w856 -> [w867] mode=indexing
          tunnel: w852 -> [w868] mode=indexing
          n318 = Build Array(w867) -> (w866:T31)
          n319 = call "Change tab page colour.vi"("Action"=T8."Change specific tabs", "New Colour"=w868, "Page Indices"=w866, "TabControl in"=w869) -> ()  [unwired: 7 in, 1 out]
        }
      }
      event "Protocol Editor": Mouse Down {
        n320 = event-data() -> ("CtlRef"=w899:refnum<vi>, "Coords"=w898:T34, "Mods.Double Click"=w900:bool)  [unwired: 1 in]
        n321 = invoke class="MCListbox (strict)" method="Point To Row Column"(reference=w899, "Point"=w898) -> (reference out=w894:refnum<vi>, error out=w893:errorcluster, "InBounds"=w885:bool, "CellPosition"=w890:T6)  [unwired: 5 in, 3 out]
        n322 = property class="MCListbox (strict)"(reference=w894, error in=w893) -> (reference out=w892:refnum<vi>, error out=w891:errorcluster, "ItemNames"=w897:string[][])
        n323 = Unbundle By Name(w890) -> ("Row"=w888:i32)
        n324 = Array Size(array=w897) -> (size(s)=w895:i32[])
        n325 = Index Array(array=w895, index=0) -> (element=w889:i32)
        n326 = Less?(x=w888, y=w889) -> (x < y?=w886:bool)
        n327 = Greater Or Equal To 0?(x=w888) -> (x >= 0?=w887:bool)
        n328 = Compound Arithmetic op=AND "Valid selection"(w885, w886, w887) -> (w884:bool)
        n329 = case shown="True" w884 {
          tunnel: w890 -> [_ w918]
          tunnel: w906 -> [_ w917]
          tunnel: [w914 w921] -> w905
          tunnel: w904 -> [w914 w922]
          tunnel: w892 -> [_ w924]
          tunnel: w891 -> [_ w923]
          tunnel: w900 -> [_ w920]
          tunnel: w883 -> [_ w916]
          tunnel: w882 -> [_ w915]
          frame False {
          }
          frame True {
            n330 = Unbundle By Name(w918) -> ("Row"=w919:i32, "Column"=w925:i32)
            n331 = case shown="Default" w925 {
              tunnel: w919 -> [_ w957 _]
              tunnel: w918 -> [w927 _ _]
              tunnel: w924 -> [w930 w947 _]
              tunnel: w923 -> [w929 w946 _]
              tunnel: w922 -> [w928 _ w964]
              tunnel: [w928 w944 w964] -> w921
              tunnel: w920 -> [w926 _ _]
              tunnel: w917 -> [_ w945 _]
              tunnel: w916 -> [_ w939 _]
              tunnel: w915 -> [_ w938 _]
              frame Default {
                n332 = case shown="False" w926 {
                  tunnel: w930 -> [w932 w937]
                  tunnel: w929 -> [w931 _]
                  tunnel: w927 -> [_ w934]
                  frame False {
                    n333 = Close Reference(reference=w932, error in (no error)=w931) -> ()  [unwired: 1 out]
                  }
                  frame True {
                    w933 = T12."Disabled and Grayed Out" ("Disabled")
                    # ">> fire an edit event == double mouse click"
                    n334 = property on="Property Node" class="MCListbox (strict)"(reference=w937, "EditPos"=w934, "ActiveCell"=w934) -> (reference out=w935:refnum<vi>, error out=w936:errorcluster)  [unwired: 1 in]
                    n335 = Close Reference(reference=w935, error in (no error)=w936) -> ()  [unwired: 1 out]
                    n336 = property on="Update waveform and Timing" class="Bool (strict)"("DisabledEnum"=w933) -> ()  [unwired: 2 in, 2 out]
                    n337 = property on="Uncage ONLY" class="Bool (strict)"("DisabledEnum"=w933) -> ()  [unwired: 2 in, 2 out]
                    n338 = property on="Uncage and Image" class="Bool (strict)"("DisabledEnum"=w933) -> ()  [unwired: 2 in, 2 out]
                  }
                }
              }
              frame 0 {
                w952 = 37
                # "update enabled stim points"
                # "1st Column (enable/disable tick box)"
                n339 = property on="Protocol Editor" class="MCListbox (strict)"() -> ("ItemSyms"=w949:i32[])  [unwired: 2 in, 2 out]
                n340 = Close Reference(reference=w947, error in (no error)=w946) -> ()  [unwired: 1 out]
                n341 = case shown="True" w945 {
                  tunnel: [w958 FALSE ("Waveform changed!")] -> w944
                  frame False {
                    w958 = TRUE  # Waveform changed!
                  }
                  frame True {
                    n342 = property on="Update waveform and Timing" class="Bool (strict)"("Val(Sgnl)"=TRUE ("Value (Signaling)")) -> ()  [unwired: 2 in, 2 out]
                  }
                }
                n343 = Index Array(array=w949, index=w957) -> (element=w950:i32)
                n344 = Equal?(x=w950, y=w952) -> (x = y?=w954:bool)
                n345 = Select(t=38, s=w954, f=w952) -> (s? t:f=w953:i32)
                n346 = Replace Array Subset(array=w949, new element=w953, index=w957) -> (w948:i32[])
                n347 = property on="Protocol Editor" class="MCListbox (strict)"("ItemSyms"=w948) -> (error out=w940:errorcluster)  [unwired: 2 in, 1 out]
                n348 = for "All enabled?" {
                  tunnel: w948 -> [w963] mode=indexing
                  tunnel: 38 -> [w962]
                  tunnel: [w961] -> w955 mode=indexing
                  n349 = Equal?(x=w963, y=w962) -> (x = y?=w961:bool)
                }
                n350 = And Array Elements(Boolean array=w955) -> (logical AND=w943:bool)
                n351 = property on="Enable/Disable All" class="Bool (strict)"("Value"=w943) -> ()  [unwired: 2 in, 2 out]
                n352 = call "Disable_stim_points_outside_stim_area.vi"("error in (no error)"=w940, "Current stim box"=w939, "Protocol Editor Ref IN"=w938) -> ("error out"=w942:errorcluster, "Protocol Editor Ref OUT"=w941:refnum<vi>)  [unwired: 7 in]
                n353 = Close Reference(reference=w941, error in (no error)=w942) -> ()  [unwired: 1 out]
              }
              frame -2, -1 {
                # "Outside the boundry (-2) or in the header (-1)"
              }
            }
          }
        }
      }
      event "Protocol Editor": Edit Cell {
        n354 = event-data() -> ("CtlRef"=w978:refnum<vi>, "String"=w972:string)  [unwired: 1 in]
        n355 = property on="Property Node" class="MCListbox (strict)"(reference=w978) -> (reference out=w976:refnum<vi>, error out=w975:errorcluster, "ActiveCell"=w977:T6)  [unwired: 1 in]
        n356 = Unbundle By Name(w977) -> ("Column"=w971:i32)
        n357 = case shown="Default" w971 {
          selector: w971 -> [w991 _ _]
          tunnel: w977 -> [w993 _ _]
          tunnel: w976 -> [w995 w1045 w1049]
          tunnel: w972 -> [w992 _ _]
          tunnel: w975 -> [w994 w1044 w1048]
          tunnel: w974 -> [w999 w1043 w1047]
          tunnel: [w998 w1043 w1047] -> w973
          tunnel: w970 -> [w997 _ _]
          tunnel: w969 -> [_ w1042 w1046]
          tunnel: [w996 w1042 w1046] -> w968
          frame Default {
            n358 = call "string test_single_cell.vi"("Column"=w991, "string"=w992) -> ("String invalid!"=w990:bool)  [unwired: 8 in]
            n359 = case "Entered string invalid?" shown="True" w990 {
              tunnel: w995 -> [w1010 w1030]
              tunnel: w993 -> [w1004 w1024]
              tunnel: [w1007 w1028] -> w989
              tunnel: w994 -> [w1009 w1029]
              tunnel: [w1006 w1027] -> w988
              tunnel: w999 -> [w1002 w1021]
              tunnel: [w1000 w1022] -> w998
              frame False {
                n360 = for "Was invalid cell ?" {
                  tunnel: w1002 -> [w1018] mode=indexing
                  tunnel: w1004 -> [w1019]
                  tunnel: [w1017] -> w1003
                  tunnel: [w1016] -> w1001
                  i -> [w1016]
                  stop <- w1017 stop-if-true
                  n361 = Equal?(x=w1019, y=w1018) -> (x = y?=w1017:bool)
                }
                n362 = property class="MCListbox (strict)"(reference=w1010, error in=w1009, "ActiveCell"=w1004, "CellBG"=u32 16777226) -> (reference out=w1007:refnum<vi>, error out=w1006:errorcluster)
                n363 = case "If so, remove it from the invalid cell array!" shown="True" w1003 {
                  tunnel: w1002 -> [w1011 w1015]
                  tunnel: w1001 -> [_ w1013]
                  tunnel: [w1011 w1012] -> w1000
                  frame False {
                  }
                  frame True {
                    n364 = Delete From Array(array=w1015, length=1, index=w1013) -> (array with subset deleted=w1012:T6[])  [unwired: 1 out]
                  }
                }
                n365 = Empty Array?(array=w1000) -> (empty?=w1005:bool)
                n366 = case shown="True" w1005 {
                  frame False {
                  }
                  frame True {
                    n367 = property on="StimModuleStatus" class="Str"("Val(Sgnl)"="" ("message")) -> ()  [unwired: 2 in, 2 out]
                  }
                }
              }
              frame True {
                n368 = Empty Array?(array=w1021) -> (empty?=w1023:bool)
                n369 = for "Known invalid cell ?" {
                  tunnel: w1021 -> [w1037] mode=indexing
                  tunnel: w1024 -> [w1038]
                  tunnel: [w1036] -> w1025
                  stop <- w1036 stop-if-true
                  n370 = Equal?(x=w1038, y=w1037) -> (x = y?=w1036:bool)
                }
                n371 = case shown="True" w1023 {
                  frame False {
                    # "The protocol is already invaild!"
                  }
                  frame True {
                    n372 = property on="StimModuleStatus" class="Str"("Val(Sgnl)"="Your protocol contains invalid values. Please correct them first!" ("message")) -> ()  [unwired: 2 in, 2 out]
                  }
                }
                n373 = property class="MCListbox (strict)"(reference=w1030, error in=w1029, "ActiveCell"=w1024, "CellBG"=u32 15663114) -> (reference out=w1028:refnum<vi>, error out=w1027:errorcluster)
                n374 = case "If not, add to list" shown="False" w1025 {
                  tunnel: w1021 -> [w1034 w1035]
                  tunnel: w1024 -> [w1033 _]
                  tunnel: [w1032 w1035] -> w1022
                  frame False {
                    n375 = Build Array (concatenate)(w1034, w1033) -> (w1032:T6[])
                  }
                  frame True {
                  }
                }
              }
            }
            n376 = Close Reference(reference=w989, error in (no error)=w988) -> ()  [unwired: 1 out]
            n377 = case shown="True" w997 {
              tunnel: [w1039 FALSE ("Waveform changed!")] -> w996
              frame False {
                w1039 = TRUE  # Waveform changed!
              }
              frame True {
                n378 = property on="Update waveform and Timing" class="Bool (strict)"("Val(Sgnl)"=TRUE ("Value (Signaling)")) -> ()  [unwired: 2 in, 2 out]
              }
            }
          }
          frame 0 {
            # "1st Column (enable/disable tick box)"
            n379 = Close Reference(reference=w1045, error in (no error)=w1044) -> ()  [unwired: 1 out]
          }
          frame -2, -1 {
            n380 = Close Reference(reference=w1049, error in (no error)=w1048) -> ()  [unwired: 1 out]
          }
        }
      }
      event "Enable/Disable All": Value Change {
        n381 = event-data() -> ("NewVal"=w1068:bool)  [unwired: 1 in]
        n382 = property class="MCListbox (strict)"(reference=w1061) -> (reference out=w1057:refnum<vi>, error out=w1056:errorcluster, "ItemSyms"=w1060:i32[])  [unwired: 1 in]
        n383 = case shown="True" w1067 {
          tunnel: [w1077 FALSE ("Waveform changed!")] -> w1066
          frame False {
            w1077 = TRUE  # Waveform changed!
          }
          frame True {
            n384 = property on="Update waveform and Timing" class="Bool (strict)"("Val(Sgnl)"=TRUE ("Value (Signaling)")) -> ()  [unwired: 2 in, 2 out]
          }
        }
        n385 = Select(t=38, s=w1068, f=37) -> (s? t:f=w1058:i32)
        n386 = Array Size(array=w1060) -> (size(s)=w1059:i32)
        n387 = Initialize Array(w1058, w1059) -> (w1055:i32[])
        n388 = property class="MCListbox (strict)"(reference=w1057, error in=w1056, "ItemSyms"=w1055) -> (reference out=w1054:refnum<vi>, error out=w1053:errorcluster)
        n389 = Close Reference(reference=w1054, error in (no error)=w1053) -> ()  [unwired: 1 out]
      }
      event "GRID": Value Change {
        # "Reso or Galvo?"
        n390 = event-data() -> ()  [unwired: 1 in, 1 out]
        n391 = flat-sequence {
          tunnel: [w1146] -> w1136
          tunnel: w1127 -> [w1146]
          frame #0 {
            n392 = property on="Protocol Editor" class="MCListbox (strict)"("ItemNames"=string[][] [] ("Item Names")) -> ()  [unwired: 2 in, 2 out]
          }
        }
        n393 = case shown="True" w1095 {
          tunnel: [w1143 FALSE ("Waveform changed!")] -> w1094
          frame False {
            w1143 = TRUE  # Waveform changed!
          }
          frame True {
            n394 = property on="Update waveform and Timing" class="Bool (strict)"("Val(Sgnl)"=TRUE ("Value (Signaling)")) -> ()  [unwired: 2 in, 2 out]
          }
        }
        n395 = call "IMAQ Clear Overlay"("Image"=w1136) -> ()  [unwired: 9 in, 2 out]
        n396 = call "IMAQ Clear Overlay"("Image"=w1101) -> ("Image Out"=w1100:T1)  [unwired: 9 in, 1 out]
        n397 = Bundle By Name(cluster=cluster{"X-Dimension":i32, "Y-Dimension":i32} {"X-Dimension"=6, "Y-Dimension"=6} ("Grid Dimensions"), "X-Dimension"="Rows", "Y-Dimension"="Columns") -> (w1124:cluster{"X-Dimension":i32, "Y-Dimension":i32})
        n398 = call-poly "GFGpolyGet.vi"("Variable Name in"="x.fov") -> ("Numeric"=w1106:dbl)  [unwired: 8 in, 2 out]
        n399 = call-poly "GFGpolyGet.vi"("Variable Name in"="y.fov") -> ("Numeric"=w1107:dbl)  [unwired: 8 in, 2 out]
        n400 = call-poly "GFGpolyGet.vi"("Variable Name in"="nomin.x.pixels") -> ("Numeric"=w1113:dbl)  [unwired: 8 in, 2 out]
        n401 = call-poly "GFGpolyGet.vi"("Variable Name in"="y.pixels") -> ("Numeric"=w1112:dbl)  [unwired: 8 in, 2 out]
        n402 = Divide(x="Grid spacing (µm)", y=1000000.0) -> (x/y=w1109:dbl)
        n403 = Bundle By Name(cluster=cluster{"Tot Y Pixels":i32, "Tot X Pixels":i32} {"Tot Y Pixels"=256, "Tot X Pixels"=256} ("Pixel Boundary (in pixels)"), "Tot X Pixels"=w1113, "Tot Y Pixels"=w1112) -> (w1111:cluster{"Tot Y Pixels":i32, "Tot X Pixels":i32})
        n404 = Bundle By Name(cluster=T20 {"X Grid Spacing (in metres)"=5e-06, "Y Grid Spacing (in metres)"=5e-06} ("Grid Spacing (in metres)"), "X Grid Spacing (in metres)"=w1109, "Y Grid Spacing (in metres)"=w1109) -> (w1119:T20)
        n405 = Bundle By Name(cluster=T19 {"X- Offset (in pixels)"=0, "Y-Offset (in pixels)"=0} ("Pixel Offsets"), "X- Offset (in pixels)"="X postition", "Y-Offset (in pixels)"="Y position") -> (w1117:T19)
        n406 = Bundle By Name(cluster=T21 {"X FOV (in metres)"=0.0007, "Y FOV (in metres)"=0.0007} ("Field Of View (in metres)"), "X FOV (in metres)"=w1106, "Y FOV (in metres)"=w1107) -> (w1121:T21)
        n407 = call "Check if same stim and Imaging Path.vi"("System Information Cluster"=w1082) -> ("Boolean"=w1081:bool)  [unwired: 10 in]
        n408 = call "Experiment with Grid Generation.vi"("Pixel Boundary (in pixels)"=w1111, "Field Of View (in metres)"=w1121, "Pixel Offsets"=w1117, "Grid Spacing (in metres)"=w1119, "Grid Dimensions"=w1124) -> ("Array of Y coordinates"=w1134:i32[], "Array of X coordinates"=w1135:i32[])  [unwired: 4 in, 1 out]
        n409 = case shown="False" w1081 {
          selector: w1081 -> [w1139 w1142]
          tunnel: [w1141 _] -> w1087
          tunnel: w1085 -> [w1140 _]
          tunnel: [w1139 w1142] -> w1080
          frame False {
            n410 = call "getPixelMapping.vi"("Key String IN"=w1140) -> ("Rectangle"=w1141:T14)  [unwired: 5 in, 5 out]
          }
          frame True {
          }
        }
        n411 = for {
          tunnel: [w1189] -> w1133 mode=indexing
          tunnel: w1135 -> [w1168] mode=indexing
          tunnel: w1134 -> [w1174] mode=indexing
          tunnel: w1103 -> [w1176]
          tunnel: [w1175] -> w1102
          tunnel: w1098 -> [w1173]
          tunnel: w1100 -> [w1170]
          tunnel: w1099 -> [w1167]
          tunnel: w1087 -> [w1165]
          tunnel: [w1163] -> w1086 mode=indexing
          tunnel: w1080 -> [w1162]
          i -> [w1182]
          n412 = Number To Decimal String(number=w1168) -> (decimal integer string=w1186:string)  [unwired: 1 in]
          n413 = Number To Decimal String(number=w1174) -> (decimal integer string=w1184:string)  [unwired: 1 in]
          n414 = Increment(x=w1182) -> (x+1=w1181:i32)
          n415 = Number To Decimal String(number=w1181) -> (decimal integer string=w1169:string)  [unwired: 1 in]
          n416 = Add(x=w1168, y=w1167) -> (x+y=w1166:i32)
          n417 = Add(x=w1174, y=w1173) -> (x+y=w1172:i32)
          n418 = Bundle("X- Offset (in pixels)"=w1168, "Y-Offset (in pixels)"=w1174) -> (w1164:T19)  [unwired: 1 in]
          n419 = case shown="False" w1162 {
            tunnel: w1165 -> [w1196 _]
            tunnel: w1164 -> [w1195 _]
            tunnel: [w1190 38] -> w1163
            frame False {
              # "Check, if the selected stimulation point is in the boundary of the stimulatable area"
              n420 = Unbundle By Name(w1195) -> ("X- Offset (in pixels)"=w1202:i32, "Y-Offset (in pixels)"=w1201:i32)
              n421 = Unbundle By Name(w1196) -> ("Left"=w1203:i32, "Top"=w1200:i32, "Right"=w1194:i32, "Bottom"=w1199:i32)
              n422 = In Range and Coerce(upper limit=w1194, x=w1202, lower limit=w1203) -> (In Range?=w1198:bool)  [unwired: 1 out]
              n423 = In Range and Coerce(upper limit=w1199, x=w1201, lower limit=w1200) -> (In Range?=w1197:bool)  [unwired: 1 out]
              n424 = And(x=w1198, y=w1197) -> (x .and. y?=w1193:bool)
              n425 = Select(t=38, s=w1193, f=37) -> (s? t:f=w1190:i32)
            }
            frame True {
              # "Stim path = Imaging path - no bounding box required!"
            }
          }
          n426 = Bundle(w1166, w1172) -> (w1171:cluster{i32, i32})  [unwired: 1 in]
          n427 = Concatenate Strings(w1169, "[" ("string"), w1186, "," ("string"), w1184, "]" ("string")) -> (w1188:string)
          n428 = call "IMAQ Overlay Text"("Group"=w1169, "Text Color (black)"=u32 13107215, "String"=w1169, "Origin"=w1171, "Image"=w1170) -> ("Image Out"=w1179:T1)  [unwired: 5 in, 1 out]
          n429 = Bundle(w1188, w1164) -> (w1189:T35)  [unwired: 1 in]
          n430 = call "IMAQ Convert Point to ROI"("Point"=w1164) -> ("ROI Descriptor"=w1178:T30)  [unwired: 8 in, 1 out]
          n431 = call "IMAQ Overlay ROI"("Colors (Green)"=u32[] [16774186], "Group"=w1169, "Point Symbol"=w1176, "ROI Descriptor"=w1178, "Image"=w1179) -> ("Image Out"=w1175:T1)  [unwired: 5 in, 1 out]
        }
        n432 = call "IMAQ Copy Overlay"("Image Dst"=w1127, "Image Src"=w1102) -> ("Image Dst Out"=w1084:T1)  [unwired: 8 in, 1 out]
        n433 = for {
          tunnel: [w1153] -> w1129 mode=indexing
          tunnel: w1133 -> [w1149] mode=indexing
          w1148 = "%^.0p" ("format string")
          n434 = property on="Stim duration (s)" class="DigNum (strict)"() -> ("Value"=w1157:dbl)  [unwired: 2 in, 2 out]
          n435 = property on="Stim interval (s)" class="DigNum (strict)"() -> ("Value"=w1156:dbl)  [unwired: 2 in, 2 out]
          n436 = property on="Spot repetitions" class="DigNum (strict)"() -> ("Value"=w1155:dbl)  [unwired: 2 in, 2 out]
          n437 = property on="Stim Power (%)" class="Slide (strict)"() -> ("Value"=w1154:dbl)  [unwired: 2 in, 2 out]
          n438 = property on="Pre-stim settling time (s)" class="DigNum (strict)"() -> ("Value"=w1152:dbl)  [unwired: 2 in, 2 out]
          n439 = Unbundle(w1149) -> (w1150:string)  [unwired: 1 out]
          n440 = Format Into String(format string=w1148, w1157) -> (resulting string=w1161:string)  [unwired: 2 in, 1 out]
          n441 = Format Into String(format string=w1148, w1156) -> (resulting string=w1160:string)  [unwired: 2 in, 1 out]
          n442 = Format Into String(format string=w1148, w1155) -> (resulting string=w1159:string)  [unwired: 2 in, 1 out]
          n443 = Format Into String(format string=w1148, w1154) -> (resulting string=w1158:string)  [unwired: 2 in, 1 out]
          n444 = Format Into String(format string=w1148, w1152) -> (resulting string=w1151:string)  [unwired: 2 in, 1 out]
          n445 = Build Array(w1150, w1161, w1160, w1159, w1158, w1151) -> (w1153:string[])
        }
        n446 = call "IMAQ Copy Overlay"("Image Dst"=w1084, "Image Src"=w1083) -> ()  [unwired: 8 in, 2 out]
        n447 = property on="Protocol Editor" class="MCListbox (strict)"("ItemNames"=w1129, "ItemSyms"=w1086) -> ()  [unwired: 2 in, 2 out]
        n448 = global write "save ROI.vi" "Save Coordinates"(w1133) -> ()
      }
      event "Update waveform and Timing": Value Change {
        # "Is there a valid calibration key\nor\nis calibration not required? (same I and S Path)"
        n449 = event-data() -> ("NewVal"=w1217:bool)  [unwired: 1 in]
        n450 = Empty String/Path?(string/path=w1209) -> (empty?=w1213:bool)
        n451 = Not(x=w1213) -> (.not. x?=w1212:bool)
        n452 = Or(x=w1212, y=w1211) -> (x .or. y?=w1210:bool)
        n453 = And(x=w1217, y=w1210) -> (x .and. y?=w1214:bool)
        n454 = case shown="True" w1214 {
          tunnel: [w1228 w1240] -> w1227
          tunnel: w1226 -> [w1228 w1239]
          tunnel: w1224 -> [_ w1238]
          tunnel: [w1229 w1237] -> w1221
          tunnel: w1220 -> [w1229 w1236]
          tunnel: w1211 -> [_ w1232]
          tunnel: w1209 -> [_ w1231]
          tunnel: w1208 -> [_ w1230]
          frame False {
          }
          frame True {
            n455 = property on="Protocol Editor" class="MCListbox (strict)"() -> ("ItemNames"=w1234:string[][], "ItemSyms"=w1235:i32[])  [unwired: 2 in, 2 out]
            n456 = Empty Array?(array=w1234) -> (empty?=w1233:bool)
            n457 = case shown="False" w1233 {
              tunnel: w1235 -> [w1241 _]
              tunnel: w1234 -> [w1242 _]
              tunnel: [w1251 w1330] -> w1240
              tunnel: w1239 -> [w1249 w1330]
              tunnel: w1238 -> [w1250 _]
              tunnel: [w1248 w1329] -> w1237
              tunnel: w1236 -> [w1247 w1329]
              tunnel: w1232 -> [w1246 _]
              tunnel: w1231 -> [w1245 _]
              tunnel: w1230 -> [w1244 _]
              frame False {
                n458 = Empty Array?(array=w1244) -> (empty?=w1243:bool)
                n459 = case shown="True" w1243 {
                  tunnel: w1242 -> [_ w1258]
                  tunnel: [-1 w1281] -> w1251
                  tunnel: w1250 -> [_ _]
                  tunnel: w1249 -> [_ w1281]
                  tunnel: [w1254 w1269] -> w1248
                  tunnel: w1247 -> [w1254 _]
                  tunnel: w1246 -> [_ w1260]
                  tunnel: w1245 -> [_ w1259]
                  tunnel: w1241 -> [_ w1257]
                  frame False {
                    n460 = disable-structure shown="Disabled" {
                      frame Disabled {
                        w1255 = FALSE
                        n461 = property on="Uncage and Image" class="Bool (strict)"("Value"=w1255) -> ()  [unwired: 2 in, 2 out]
                        n462 = property on="Uncage ONLY" class="Bool (strict)"("Value"=w1255) -> ()  [unwired: 2 in, 2 out]
                      }
                      frame Enabled {
                      }
                    }
                    n463 = property on="Update waveform and Timing" class="Bool (strict)"("Value"=FALSE ("Value (Signaling)")) -> ()  [unwired: 2 in, 2 out]
                  }
                  frame True {
                    w1269 = FALSE  # Waveform updated - No change!
                    w1298 = T36 {"AO samp rate_XY (samples/s)"=100000.0, "AO samp rate_Pockels (samples/s)"=100000.0, "DO samp rate_Gate (samples/s)"=100000.0}  # Sampling Rates
                    w1266 = 100000.0  # DO samp rate_Gate (samples/s)
                    w1264 = 100000.0  # AO samp rate_Pockels (samples/s)
                    w1265 = 100000.0  # AO samp rate_XY (samples/s)
                    n464 = for "Only use activated stim points" {
                      tunnel: w1258 -> [w1300] mode=indexing
                      tunnel: w1257 -> [w1301] mode=indexing
                      tunnel: [w1300] -> w1256 mode=indexing if=w1299
                      n465 = Equal?(x=w1301, y=38) -> (x = y?=w1299:bool)
                    }
                    n466 = call "Stim prot to numeric array.vi"("Calibration Key"=w1259, "Skip Pixel Mapping? (Same I/S Path)"=w1260, "Stm Protocol"=w1256) -> ("Stim Array (with voltage) OUT"=w1296:T37[])  [unwired: 8 in]
                    n467 = property on="Group reps" class="DigNum (strict)"() -> ("Value"=w1292:dbl)  [unwired: 2 in, 2 out]
                    n468 = property on="Rep interval (s)" class="DigNum (strict)"() -> ("Value"=w1291:dbl)  [unwired: 2 in, 2 out]
                    n469 = property on="Pre-Stim Baseline" class="DigNum (strict)"() -> ("Value"=w1285:dbl)  [unwired: 2 in, 2 out]
                    n470 = Bundle By Name(cluster=T23 {"Group repetitions"=0, "Repetition Interval"=0.0, "Pre-stim baseline"=0.0} ("Group Parameters"), "Group repetitions"=w1292, "Repetition Interval"=w1291, "Pre-stim baseline"=w1285) -> (w1293:T23)
                    n471 = property on="Pre-stim baseline (s)" class="Bool (strict)"() -> ("Value"=w1288:bool)  [unwired: 2 in, 2 out]
                    n472 = property on="Wait for external trigger" class="Bool (strict)"() -> ("Value"=w1287:bool)  [unwired: 2 in, 2 out]
                    n473 = Bundle By Name(cluster=w1298, "AO samp rate_XY (samples/s)"=w1265, "AO samp rate_Pockels (samples/s)"=w1264, "DO samp rate_Gate (samples/s)"=w1266) -> (w1297:T36)
                    n474 = Bundle By Name(cluster=T22 {"Pre-stim Wait"=FALSE, "Wait for external trigger"=FALSE} ("Trigger Parameters"), "Pre-stim Wait"=w1288, "Wait for external trigger"=w1287) -> (w1286:T22)
                    n475 = flat-sequence {
                      tunnel: w1286 -> [w1304]
                      tunnel: w1293 -> [w1305]
                      tunnel: w1296 -> [w1306]
                      tunnel: w1297 -> [w1307]
                      tunnel: [w1307] -> w1280
                      tunnel: [w1306] -> w1279
                      tunnel: [w1305] -> w1278
                      tunnel: [w1304] -> w1277
                      tunnel: [w1303] -> w1263
                      tunnel: [w1316] -> w1294
                      tunnel: [w1314] -> w1290
                      tunnel: w1280 -> [w1318]
                      tunnel: w1279 -> [w1317]
                      tunnel: w1278 -> [w1315]
                      tunnel: w1277 -> [w1313]
                      tunnel: [w1312] -> w1276
                      tunnel: [w1311] -> w1275
                      tunnel: [w1310] -> w1274
                      tunnel: [w1309] -> w1273
                      tunnel: w1263 -> [w1308]
                      tunnel: [w1308] -> w1262
                      tunnel: [w1322] -> w1282
                      tunnel: [w1323] -> w1283
                      tunnel: [w1324] -> w1270
                      tunnel: [w1325] -> w1284
                      tunnel: w1276 -> [w1325]
                      tunnel: w1275 -> [w1324]
                      tunnel: w1274 -> [w1323]
                      tunnel: w1273 -> [w1322]
                      tunnel: [w1321] -> w1272
                      tunnel: [errorcluster {"status"=FALSE, "code"=0, "source"=""} ("error constant")] -> w1267
                      tunnel: w1262 -> [w1319]
                      tunnel: [w1319] -> w1261
                      frame #0 {
                        n476 = Tick Count (ms)() -> (millisecond timer value=w1303:u32)
                        n477 = call <vilib>:"Set Busy.vi"() -> ()  [unwired: 10 in, 2 out]
                      }
                      frame #1 {
                        n478 = call "Experiment with Waveform Generation.vi"("Stim Points Array IN"=w1317, "Trigger Parameters"=w1313, "Sampling Rates"=w1318, "Group Parameters"=w1315) -> ("Group Duration (Seconds)"=w1314:dbl, "Gate Wavefprm (digital)"=w1311:digitalwaveform, "XY Waveform"=w1310:waveform(dbl)[], "Pockels Waveform"=w1309:waveform(dbl), "Total Protocol Time (s)"=w1316:dbl, "Stim Waveform Graph"=w1312:waveform(dbl)[])  [unwired: 2 in]
                      }
                      frame #2 {
                        n479 = Tick Count (ms)() -> (millisecond timer value=w1321:u32)
                        n480 = call <vilib>:"Unset Busy.vi"() -> ()  [unwired: 11 in, 1 out]
                      }
                    }
                    n481 = Subtract(x=w1272, y=w1261) -> (x-y=→"Time for generating waveforms (ms)":u32)
                    n482 = property on="Update waveform and Timing" class="Bool (strict)"(error in=w1267, "Value"=FALSE ("Value (Signaling)")) -> ()  [unwired: 1 in, 2 out]
                    n483 = global write "Global Variable_Waveforms.vi" "Pockels Waveform"(w1282) -> ()
                    n484 = global write "Global Variable_Waveforms.vi" "XY Waveform"(w1283) -> ()
                    n485 = global write "Global Variable_Waveforms.vi" "Gate Wavefprm (digital)"(w1270) -> ()
                    n486 = property on="Group Duration (s)" class="DigNum (strict)"("Value"=w1290) -> ()  [unwired: 2 in, 2 out]
                    n487 = property on="Total time (s)" class="DigNum (strict)"("Value"=w1294) -> ()  [unwired: 2 in, 2 out]
                    "Waveform Graph" <- w1284
                  }
                }
              }
              frame True {
                w1326 = 0.0
                w1328 = FALSE
                n488 = disable-structure shown="Disabled" {
                  frame Disabled {
                    n489 = One Button Dialog(message="Select at least one stimulation point!") -> ()  [unwired: 1 in, 1 out]
                  }
                  frame Enabled {
                  }
                }
                n490 = property on="Uncage ONLY" class="Bool (strict)"("Value"=w1328) -> ()  [unwired: 2 in, 2 out]
                n491 = property on="Uncage and Image" class="Bool (strict)"("Value"=w1328) -> ()  [unwired: 2 in, 2 out]
                n492 = property on="Update waveform and Timing" class="Bool (strict)"("Value"=w1328) -> ()  [unwired: 2 in, 2 out]
                n493 = property on="Waveform Graph" class="WFGraph (strict)"("Value"=waveform(dbl)[] [] ("Waveform Graph")) -> ()  [unwired: 2 in, 2 out]
                n494 = property on="Total time (s)" class="DigNum (strict)"("Value"=w1326) -> ()  [unwired: 2 in, 2 out]
                n495 = property on="Group Duration (s)" class="DigNum (strict)"("Value"=w1326) -> ()  [unwired: 2 in, 2 out]
              }
            }
          }
        }
      }
      event "StimModuleStatus": Value Change {
        # "Empty calibration\nand NOT\nCalibration NOT required"
        n496 = event-data() -> ("OldVal"=w1342:string, "NewVal"=w1343:string)  [unwired: 1 in]
        n497 = Not(x=w1333) -> (.not. x?=w1332:bool)
        n498 = Empty Array?(array=w1341) -> (empty?=w1340:bool)
        n499 = Empty String/Path?(string/path=w1339) -> (empty?=w1338:bool)
        n500 = And(x=w1338, y=w1332) -> (x .and. y?=w1334:bool)
        n501 = case shown="\"\", Default" w1343 {
          tunnel: w1342 -> [_ _ _ _]
          tunnel: w1340 -> [w1356 w1358 _ w1368]
          tunnel: w1334 -> [_ _ w1366 w1367]
          frame "Calibration unavailable for current scanner settings! Click on 'Calibrate' to start" {
            w1354 = T12."Disabled and Grayed Out" ("Disabled")
            n502 = Select(t=T12."Enabled" ("Disabled"), s=w1356, f=w1354) -> (s? t:f=w1353:T12)
            n503 = property on="Image1" class="ImageControl"("DisabledEnum"=w1354) -> ()  [unwired: 2 in, 2 out]
            n504 = property on="Uncage ONLY" class="Bool (strict)"("DisabledEnum"=w1354) -> ()  [unwired: 2 in, 2 out]
            n505 = property on="Uncage and Image" class="Bool (strict)"("DisabledEnum"=w1354) -> ()  [unwired: 2 in, 2 out]
            n506 = property on="Update waveform and Timing" class="Bool (strict)"("DisabledEnum"=w1353) -> ()  [unwired: 2 in, 2 out]
            n507 = property on="Calibrate" class="Bool"("Blinking"=TRUE) -> ()  [unwired: 2 in, 2 out]
          }
          frame "Cannot mark stim points on a Line Scan image!" {
            n508 = disable-structure shown="Enabled" {
              disable-tunnel: w1358 -> [w1362 _]
              frame Enabled {
                w1360 = T12."Disabled and Grayed Out" ("Disabled")
                n509 = Select(t=T12."Enabled" ("Disabled"), s=w1362, f=w1360) -> (s? t:f=w1359:T12)
                n510 = property on="Image1" class="ImageControl"("DisabledEnum"=w1360) -> ()  [unwired: 2 in, 2 out]
                n511 = property on="Update waveform and Timing" class="Bool (strict)"("DisabledEnum"=w1359) -> ()  [unwired: 2 in, 2 out]
              }
              frame Disabled {
              }
            }
          }
          frame "Your protocol contains invalid values. Please correct them first!" {
            w1365 = T12."Disabled and Grayed Out" ("Disabled")
            n512 = Select(t=w1365, s=w1366, f=T12."Enabled" ("Disabled")) -> (s? t:f=w1363:T12)
            n513 = property on="Image1" class="ImageControl"("DisabledEnum"=w1363) -> ()  [unwired: 2 in, 2 out]
            n514 = property on="Uncage ONLY" class="Bool (strict)"("DisabledEnum"=w1365) -> ()  [unwired: 2 in, 2 out]
            n515 = property on="Uncage and Image" class="Bool (strict)"("DisabledEnum"=w1365) -> ()  [unwired: 2 in, 2 out]
            n516 = property on="Update waveform and Timing" class="Bool (strict)"("DisabledEnum"=w1365) -> ()  [unwired: 2 in, 2 out]
            n517 = property on="Calibrate" class="Bool"("Blinking"=w1366) -> ()  [unwired: 2 in, 2 out]
          }
          frame "", Default {
            n518 = case shown="True" w1368 {
              tunnel: w1367 -> [w1369 w1371]
              frame False {
                n519 = case shown="False" w1369 {
                  frame False {
                    # "Still invalid protocol!"
                    n520 = property on="StimModuleStatus" class="Str"("Val(Sgnl)"="Your protocol contains invalid values. Please correct them first!" ("Variable Name in")) -> ()  [unwired: 2 in, 2 out]
                  }
                  frame True {
                    # "Error in protocol and calibration. This case should not exsist."
                  }
                }
              }
              frame True {
                n521 = case shown="False" w1371 {
                  frame False {
                    w1372 = T12."Enabled" ("Disabled")
                    # "No more errors."
                    n522 = property on="Image1" class="ImageControl"("DisabledEnum"=w1372) -> ()  [unwired: 2 in, 2 out]
                    n523 = property on="Uncage ONLY" class="Bool (strict)"("DisabledEnum"=w1372) -> ()  [unwired: 2 in, 2 out]
                    n524 = property on="Uncage and Image" class="Bool (strict)"("DisabledEnum"=w1372) -> ()  [unwired: 2 in, 2 out]
                    n525 = property on="Update waveform and Timing" class="Bool (strict)"("DisabledEnum"=w1372) -> ()  [unwired: 2 in, 2 out]
                    n526 = property on="Calibrate" class="Bool"("Blinking"=FALSE) -> ()  [unwired: 2 in, 2 out]
                  }
                  frame True {
                    # "Still not calibrated!"
                    n527 = property on="StimModuleStatus" class="Str"("Val(Sgnl)"="Calibration unavailable for current scanner settings! Click on 'Calibrate' to start" ("Variable Name in")) -> ()  [unwired: 2 in, 2 out]
                  }
                }
              }
            }
          }
        }
      }
      event "Auto Update?": Value Change {
        # "Ensure that the Auto update control/tunnel has the up to date value"
        n528 = event-data() -> ()  [unwired: 1 in, 1 out]
      }
      event "Uncage ONLY", "Uncage and Image": Value Change {
        n529 = event-data() -> ("NewVal"=w1403:bool)  [unwired: 1 in]
        n530 = case shown="True" w1403 {
          tunnel: [refnum<k21> refnum ("task out") w1443] -> w1409
          tunnel: [refnum<k21> refnum ("task out") w1442] -> w1408
          tunnel: [-1 w1441] -> w1407
          tunnel: w1406 -> [_ w1436]
          tunnel: w1405 -> [w1418 w1438]
          tunnel: w1404 -> [w1417 w1437]
          tunnel: [FALSE ("Value") w1435] -> w1401
          tunnel: w1400 -> [_ w1434]
          tunnel: [refnum<k21> refnum ("Pockels and Piezo Task OUT") w1433] -> w1399
          tunnel: w1398 -> [w1413 w1432]
          tunnel: w1397 -> [_ w1431]
          tunnel: [_ w1430] -> w1395
          tunnel: w1389 -> [w1410 w1429]
          frame False {
            w1416 = T12."Enabled" ("Disabled")
            # "Cancel Uncaging - So  clear the tasks"
            n531 = call <vilib>:"DAQmx Clear Task.vi"("task in"=w1413) -> ()  [unwired: 14 in, 1 out]
            n532 = flat-sequence {
              frame #0 {
                # "Park mirror"
                n533 = call "reset AO_galvo_stim.vi"() -> ()  [unwired: 11 in, 1 out]
              }
              frame #1 {
                n534 = property on="Uncaging Shutter" class="Bool (strict)"("Val(Sgnl)"=FALSE ("Value (Signaling)")) -> ()  [unwired: 2 in, 2 out]
              }
            }
            n535 = case "If same Stim and Im Path; reset Pockels voltage to the last scan voltage set by the user from SciScan GUI" shown="True" w1410 {
              frame False {
              }
              frame True {
                (unwired) 0.0 ("Numeric")
                w1424 = "Laser.Power" ("Variable Name in")
                n536 = call "GFGnumericGet.vi"("Variable Name in"=w1424) -> ("error out"=w1423:errorcluster, "Numeric"=w1422:dbl)  [unwired: 8 in, 1 out]
                n537 = call "GFG_core.vi"("Variable Name in"=w1424, "Variant in"=w1422, "error in (no error)"=w1423, "Action"=enum16{"Init", "Set", "Get", "Clear"}."Set") -> ()  [unwired: 9 in, 7 out]
              }
            }
            n538 = call <vilib>:"DAQmx Clear Task.vi"("task in"=w1417) -> ()  [unwired: 14 in, 1 out]
            n539 = call <vilib>:"DAQmx Clear Task.vi"("task in"=w1418) -> ()  [unwired: 14 in, 1 out]
            n540 = property on="Uncage ONLY" class="Bool (strict)"("DisabledEnum"=w1416) -> ()  [unwired: 2 in, 2 out]
            n541 = property on="Uncage and Image" class="Bool (strict)"("DisabledEnum"=w1416) -> ()  [unwired: 2 in, 2 out]
            n542 = call-poly "GFGpolyGet.vi"("Variable Name in"="Hyperscope.type") -> ("String"=w1411:string)  [unwired: 9 in, 1 out]
            n543 = case "Special Case for RGG where Pockels sits on PCI 6110" shown="\"RGG\"" w1411 {
              frame "False", Default {
              }
              frame "RGG" {
                n544 = call "Timebase and Trigger Routing.vi"("Signal Router Action"=Timebase_and_Trigger_Routing."Disconnect all", "System Type"="Stimulation Only (RGG Case)" ("Variable Name in")) -> ()  [unwired: 9 in, 1 out]
              }
            }
          }
          frame True {
            n545 = property on="Protocol Editor" class="MCListbox (strict)"() -> ("ItemNames"=w1439:string[][])  [unwired: 2 in, 2 out]
            n546 = Empty Array?(array=w1439) -> (empty?=w1440:bool)
            n547 = case shown="False" w1440 {
              tunnel: [w1452 w1536] -> w1443
              tunnel: [w1451 w1537] -> w1442
              tunnel: [w1450 w1535] -> w1441
              tunnel: w1438 -> [_ w1536]
              tunnel: w1437 -> [_ w1537]
              tunnel: w1436 -> [_ w1535]
              tunnel: [w1449 FALSE ("Value")] -> w1435
              tunnel: w1434 -> [w1448 _]
              tunnel: [w1447 w1532] -> w1433
              tunnel: w1432 -> [_ w1532]
              tunnel: w1431 -> [w1446 _]
              tunnel: [w1445 _] -> w1430
              tunnel: w1429 -> [w1444 _]
              frame False {
                n548 = case shown="False" w1446 {
                  tunnel: [w1472 -1] -> w1450
                  tunnel: [w1468 _] -> w1452
                  tunnel: [w1465 _] -> w1451
                  tunnel: [w1460 w1530] -> w1449
                  tunnel: [w1458 _] -> w1447
                  tunnel: w1448 -> [_ w1530]
                  tunnel: ["stim in progress" ("Variable Name in") _] -> w1445
                  tunnel: w1444 -> [w1453 _]
                  frame False {
                    n549 = global read "Global Variable_Waveforms.vi" "Pockels Waveform"() -> (w1464:waveform(dbl))
                    n550 = global read "Global Variable_Waveforms.vi" "XY Waveform"() -> (w1463:waveform(dbl)[])
                    n551 = global read "Global Variable_Waveforms.vi" "Gate Wavefprm (digital)"() -> (w1459:digitalwaveform)
                    n552 = property on="Uncage ONLY" class="Bool (strict)"() -> ("Value"=w1460:bool)  [unwired: 2 in, 2 out]
                    n553 = property on="Uncage and Image" class="Bool (strict)"() -> ("Value"=w1455:bool)  [unwired: 2 in, 2 out]
                    n554 = disable-structure shown="Enabled" {
                      disable-tunnel: [w1479 w1488] -> w1457
                      disable-tunnel: w1455 -> [w1478 _]
                      disable-tunnel: w1453 -> [_ w1488]
                      frame Enabled {
                        n555 = call-poly "GFGpolyGet.vi"("Variable Name in"="Hyperscope") -> ("Boolean Value OUT"=w1476:bool)  [unwired: 9 in, 1 out]
                        n556 = call-poly "GFGpolyGet.vi"("Variable Name in"="scanner.type") -> ("String"=w1483:string)  [unwired: 9 in, 1 out]
                        n557 = call-poly "GFGpolyGet.vi"("Variable Name in"="Hyperscope.type") -> ("String"=w1486:string)  [unwired: 9 in, 1 out]
                        n558 = Not(x=w1476) -> (.not. x?=w1475:bool)
                        n559 = Equal?(x="Stimulation Path Galvo", y=w1483) -> (x = y?=w1480:bool)
                        n560 = Equal?(x=w1486, y="RGG") -> (x = y?=w1481:bool)
                        n561 = Compound Arithmetic op=OR(w1478, w1481, w1480, w1475) -> (w1479:bool)
                      }
                      frame Disabled {
                        # "Code Cleanup --Arjun 19/05 /2017\n\nThe check for \"Stim path == Im path\"\nhas been implemented in a a subVI.\n\n*No need to run the check again; just use the available boolean value instead\n* It is pointless to check is an Uncage and Image - This option should be hidden away in this scenario"
                      }
                    }
                    n562 = property on="Wait for external trigger" class="Bool (strict)"() -> ("Value"=w1461:bool)  [unwired: 2 in, 2 out]
                    n563 = case "Cancel any Focus before stimulation if: <not hyperscope>,<RGG type>, <Stim Path Galvo>" shown="True" w1457 {
                      tunnel: [_ w1490] -> w1456
                      frame False {
                      }
                      frame True {
                        n564 = flat-sequence {
                          tunnel: [w1492] -> w1489
                          tunnel: [w1495] -> w1490
                          tunnel: w1489 -> [w1495]
                          frame #0 {
                            n565 = call "GFG_core.vi"("Variable Name in"="Cancel", "Variant in"=TRUE, "Action"=enum16{"Init", "Set", "Get", "Clear"}."Set") -> ("error out"=w1492:errorcluster)  [unwired: 10 in, 6 out]
                          }
                          frame #1 {
                            w1496 = u32 6000  # timeout
                            n566 = Tick Count (ms)() -> (millisecond timer value=w1497:u32)
                            n567 = while {
                              tunnel: w1497 -> [w1501]
                              tunnel: w1496 -> [w1499]
                              stop <- w1507 stop-if-true
                              n568 = Tick Count (ms)() -> (millisecond timer value=w1502:u32)
                              n569 = Subtract(x=w1502, y=w1501) -> (x-y=w1500:u32)
                              n570 = call "GFGTranslator__WRAPPER.vi"("GFGTranslator Datatype"=GFGTranslator_Datatype."Boolean", "GFG Translator Action"=GFGTranslator_Action."Get", "GFG Variable Name"="scanengine_running") -> ("Boolean_Output"=w1508:bool, "Status Output"=w1505:T25)  [unwired: 3 in, 4 out]
                              n571 = Greater?(x=w1500, y=w1499) -> (0:w1498:bool)
                              n572 = Not(x=w1508) -> (.not. x?=w1503:bool)
                              n573 = Not Equal?(x=w1505, y=GFGTranslator_errors."Success" ("Status Output")) -> (x != y?=w1504:bool)
                              n574 = Compound Arithmetic op=OR(w1504, w1503, w1498) -> (w1507:bool)
                              n575 = Wait (ms)(milliseconds to wait=u32 200) -> ()  [unwired: 1 out]
                            }
                          }
                        }
                      }
                    }
                    n576 = Select(t=UncageType."Uncage & Image", s=w1455, f=UncageType."Uncage Only" ("Uncage Type")) -> (s? t:f=w1469:T24)
                    n577 = case shown="False" w1455 {
                      frame False {
                        n578 = property on="Uncage and Image" class="Bool (strict)"("DisabledEnum"=T12."Disabled and Grayed Out" ("Disabled")) -> ()  [unwired: 2 in, 2 out]
                      }
                      frame True {
                        n579 = property on="Uncage ONLY" class="Bool (strict)"("DisabledEnum"=T12."Disabled and Grayed Out" ("Disabled")) -> ()  [unwired: 2 in, 2 out]
                      }
                    }
                    n580 = flat-sequence {
                      tunnel: w1464 -> [w1515]
                      tunnel: w1463 -> [w1516]
                      tunnel: [w1516] -> w1474
                      tunnel: [w1515] -> w1473
                      tunnel: w1456 -> [_]
                      tunnel: [w1518] -> w1467
                      tunnel: [w1517] -> w1466
                      tunnel: w1474 -> [w1517]
                      tunnel: w1473 -> [w1518]
                      frame #0 {
                        # "Park mirrors before opening shutter"
                        n581 = call "reset AO_galvo_stim.vi"() -> ()  [unwired: 11 in, 1 out]
                      }
                      frame #1 {
                        n582 = property on="Uncaging Shutter" class="Bool (strict)"("Val(Sgnl)"=TRUE ("Value (Signaling)")) -> ()  [unwired: 2 in, 2 out]
                      }
                    }
                    n583 = call "Configure Uncaging.vi"("external trigger enabled? (Uncage ONLY)"=w1461, "Uncage Type"=w1469, "Gate Waveform (Digital)"=w1459, "Pockels Waveform"=w1467, "XY Waveform"=w1466) -> ("Gate Task OUT"=w1458:refnum<k21>, "Pockels Task OUT"=w1465:refnum<k21>, "XY Mirror voltage Task OUT"=w1468:refnum<k21>)  [unwired: 4 in]
                    n584 = call "Query if Galvo or Reso.vi"() -> ("System Type"=w1462:enum16{"Galvo", "Reso"})  [unwired: 10 in, 1 out]
                    n585 = case shown="\"Reso\"" w1462 {
                      tunnel: [20 20] -> w1472
                      frame "Galvo", Default {
                      }
                      frame "Reso" {
                      }
                    }
                    n586 = case shown="\"Uncage & Image\"" w1469 {
                      tunnel: w1465 -> [_ _]
                      frame "Uncage Only", Default {
                      }
                      frame "Uncage & Image" {
                        n587 = call-poly "GFGpolyGet.vi"("Variable Name in"="Record") -> ("output cluster"=w1525:T38)  [unwired: 9 in, 1 out]
                        n588 = Unbundle By Name(w1525) -> ("BooleanRef"=w1524:refnum<vi>)
                        n589 = property class="Bool"(reference=w1524, "Val(Sgnl)"=TRUE) -> (reference out=w1521:refnum<vi>, error out=w1522:errorcluster)  [unwired: 1 in]
                        n590 = Close Reference(reference=w1521, error in (no error)=w1522) -> ()  [unwired: 1 out]
                      }
                    }
                  }
                  frame True {
                    w1528 = FALSE
                    n591 = property on="Uncage and Image" class="Bool (strict)"("Value"=w1528) -> ()  [unwired: 2 in, 2 out]
                    n592 = property on="Uncage ONLY" class="Bool (strict)"("Value"=w1528) -> ()  [unwired: 2 in, 2 out]
                    n593 = One Button Dialog(message="Please press \"Build Waveform & Estimate Timing\" button first!") -> ()  [unwired: 1 in, 1 out]
                  }
                }
              }
              frame True {
                w1534 = FALSE
                n594 = property on="Uncage ONLY" class="Bool (strict)"("Value"=w1534) -> ()  [unwired: 2 in, 2 out]
                n595 = property on="Uncage and Image" class="Bool (strict)"("Value"=w1534) -> ()  [unwired: 2 in, 2 out]
                n596 = One Button Dialog(message="Select at least one stimulation point!") -> ()  [unwired: 1 in, 1 out]
              }
            }
          }
        }
      }
      event "Save Stim Protocol": Value Change {
        n597 = event-data() -> ()  [unwired: 1 in, 1 out]
        n598 = property on="Protocol Editor" class="MCListbox (strict)"() -> ("ItemNames"=w1552:string[][])  [unwired: 2 in, 2 out]
        n599 = Empty Array?(array=w1552) -> (empty?=w1551:bool)
        n600 = case shown="False" w1551 {
          tunnel: w1552 -> [w1558 _]
          tunnel: w1549 -> [w1556 _]
          frame False {
            n601 = disable-structure shown="Enabled" {
              disable-tunnel: w1558 -> [w1564 _]
              disable-tunnel: [w1562 TRUE] -> w1557
              disable-tunnel: w1556 -> [w1561 _]
              frame Disabled {
                n602 = flat-sequence {
                  tunnel: w1561 -> [_]
                  frame #0 {
                    n603 = property on="Protocol Editor" class="MCListbox (strict)"("Value"=i32[] [] ("Stimulation Protocol")) -> ()  [unwired: 2 in, 2 out]
                  }
                }
                n604 = call "string test.vi"("Array"=w1564) -> ("Modified Array Out"=w1559:dbl[], "Location"=w1563:i32[][])  [unwired: 9 in]
                n605 = Empty Array?(array=w1559) -> (empty?=w1560:bool)
                n606 = case shown="False" w1560 {
                  tunnel: w1563 -> [w1566 _]
                  tunnel: w1561 -> [_ _]
                  tunnel: [FALSE TRUE] -> w1562
                  frame False {
                    n607 = for {
                      tunnel: w1566 -> [w1572] mode=indexing
                      n608 = Index Array(array=w1572, index=0) -> (element=w1573:i32)
                      n609 = Index Array(array=w1572, index=1) -> (element=w1570:i32)
                      n610 = Not Equal To 0?(x=w1570) -> (x != 0?=w1569:bool)
                      n611 = case shown="True" w1569 {
                        tunnel: w1573 -> [_ w1578]
                        tunnel: w1570 -> [_ w1577]
                        frame False {
                        }
                        frame True {
                          n612 = Bundle By Name(cluster=T6 {"Row"=0, "Column"=0} ("Active Cell:Active Cell"), "Row"=w1578, "Column"=w1577) -> (w1576:T6)
                          n613 = property on="Protocol Editor" class="MCListbox (strict)"("ActiveCell"=w1576, "CellBG"=u32 15663114) -> ()  [unwired: 2 in, 2 out]
                        }
                      }
                    }
                    n614 = One Button Dialog(message="Stim Points is not saved , Please enter the valid value") -> ()  [unwired: 1 in, 1 out]
                  }
                  frame True {
                  }
                }
              }
              frame Enabled {
                # "Let the user write wrong protocols."
              }
            }
            n615 = case shown="True" w1557 {
              frame False {
              }
              frame True {
                n616 = control-ref of="Protocol Editor"() -> (w1586:refnum<vi>)
                n617 = call-poly "GFGpolyGet.vi"("Variable Name in"="root.path") -> ("Path"=w1585:path)  [unwired: 8 in, 2 out]
                n618 = call "save stim points.vi"("Stim ref"=w1586, "File Name"="Protocol Name", "path"=w1585) -> ("new file path (Not A Path if cancelled)"=w1584:path)  [unwired: 8 in]
                n619 = call <vilib>:"Get File Extension.vi"("file"=w1584) -> ("filename without extension"=w1582:string)  [unwired: 7 in, 3 out]
                n620 = property on="Protocol Name" class="Str"("Value"=w1582) -> ()  [unwired: 2 in, 2 out]
              }
            }
          }
          frame True {
            n621 = One Button Dialog(message="Stim Protocol is empty, cannot save the file") -> ()  [unwired: 1 in, 1 out]
          }
        }
      }
      event "Load Stim Protocol": Value Change {
        n622 = event-data() -> ()  [unwired: 1 in, 1 out]
        n623 = call-poly "GFGpolyGet.vi"("Variable Name in"="root.path") -> ("Path"=w1602:path)  [unwired: 8 in, 2 out]
        n624 = Build Path(base path=w1602, name or relative path="Stim Protocols") -> (appended path=w1612:path)
        n625 = Path To String(path=w1612) -> (string=w1610:string)
        n626 = Concatenate Strings(w1610, "\\") -> (w1609:string)
        n627 = String To Path(string=w1609) -> (path=w1608:path)
        n628 = call "File Dialog"("start path"=w1608, "pattern (all files)"="*.stm") -> ("selected path"=w1620:path, "cancelled"=w1619:bool, "error out"=w1618:errorcluster)  [unwired: 10 in, 1 out]
        n629 = call <vilib>:"Clear Errors.vi"("error in (no error)"=w1618) -> ()  [unwired: 6 in, 1 out]
        n630 = case shown="False" w1619 {
          tunnel: w1620 -> [w1649 _]
          tunnel: [w1640 w1723] -> w1599
          tunnel: w1598 -> [_ w1723]
          tunnel: w1597 -> [w1638 _]
          tunnel: w1596 -> [w1628 _]
          tunnel: w1595 -> [w1637 _]
          tunnel: w1594 -> [w1636 _]
          tunnel: w1590 -> [w1631 _]
          tunnel: w1589 -> [w1625 _]
          frame False {
            # "discard whole stim point overlay"
            # "discard whole overlay"
            # "Update Protocol Editor"
            # "copy new stim point overlay"
            # "redraw the bounding box"
            n631 = call <vilib>:"Get File Extension.vi"("file"=w1649) -> ("filename without extension"=w1648:string)  [unwired: 7 in, 3 out]
            n632 = call "IMAQ Clear Overlay"("Image"=w1637) -> ("Image Out"=w1623:T1)  [unwired: 9 in, 1 out]
            n633 = call "IMAQ Clear Overlay"("Image"=w1638) -> ("Image Out"=w1621:T1)  [unwired: 9 in, 1 out]
            n634 = property on="Protocol Name" class="Str"("Value"=w1648) -> ()  [unwired: 2 in, 2 out]
            n635 = call-poly <vilib>:"Read From Spreadsheet File.vi"("delimiter (\\t)"=";" ("delimiter (\\t)"), "transpose (no:F)"=TRUE, "file path (dialog if empty)"=w1649) -> ("all rows"=w1658:string[][])  [unwired: 4 in, 4 out]
            n636 = Transpose 2D Array(2D array=w1658) -> (transposed array=w1655:string[][])
            n637 = Array Subset(array=w1655, index (row)=1 ("index")) -> (w1652:string[][])  [unwired: 3 in]
            n638 = call "Check if same stim and Imaging Path.vi"("System Information Cluster"=w1625) -> ("Boolean"=w1626:bool)  [unwired: 10 in]
            n639 = Delete From Array(array=w1652, index (col)=0 ("disabled index (col)")) -> (deleted portion=w1650:string[], array with subset deleted=w1646:string[][])  [unwired: 2 in]
            n640 = case shown="False" w1626 {
              selector: w1626 -> [w1660 w1663]
              tunnel: [w1662 _] -> w1632
              tunnel: w1631 -> [w1661 _]
              tunnel: [w1660 w1663] -> w1624
              frame False {
                n641 = call "getPixelMapping.vi"("Key String IN"=w1661) -> ("Rectangle"=w1662:T14)  [unwired: 5 in, 5 out]
              }
              frame True {
              }
            }
            n642 = Index Array(array=w1646, index (col)=0 ("disabled index (col)")) -> (element=w1656:string[])  [unwired: 1 in]
            n643 = call "itemstring to item array.vi"("Item sym string"=w1650) -> ("Item sym"=w1630:i32[])  [unwired: 10 in]
            n644 = Array Size(array=w1646) -> (size(s)=w1645:i32[])
            n645 = Index Array(array=w1645, index=1) -> (element=w1643:i32)
            n646 = for {
              tunnel: w1656 -> [w1687] mode=indexing
              tunnel: [w1688] -> w1639 mode=indexing
              tunnel: [w1686] -> w1622
              tunnel: w1632 -> [w1683]
              tunnel: w1630 -> [w1681] mode=indexing
              tunnel: [w1682] -> w1629 mode=indexing
              tunnel: w1624 -> [w1680]
              tunnel: w1623 -> [w1677]
              w1704 = 1 ("offset (0)")
              # "Check, if the selected stimulation point is in the boundary of the stimulatable area"
              n647 = Search/Split String(string=w1687, search string/char (-)="[") -> (substring before match=w1678:string, match + rest of string=w1707:string)  [unwired: 1 in, 1 out]
              n648 = String Subset(string=w1707, offset (0)=w1704) -> (substring=w1706:string)  [unwired: 1 in]
              n649 = Reverse String(1:w1706) -> (0:w1705:string)
              n650 = String Subset(string=w1705, offset (0)=w1704) -> (substring=w1703:string)  [unwired: 1 in]
              n651 = Reverse String(1:w1703) -> (0:w1702:string)
              n652 = Search/Split String(string=w1702, search string/char (-)=",") -> (substring before match=w1698:string, match + rest of string=w1700:string)  [unwired: 1 in, 1 out]
              n653 = String Subset(string=w1700, offset (0)=1) -> (substring=w1697:string)  [unwired: 1 in]
              n654 = Decimal String To Number(string=w1698) -> (number=w1685:i32)  [unwired: 2 in, 1 out]
              n655 = Decimal String To Number(string=w1697) -> (number=w1684:i32)  [unwired: 2 in, 1 out]
              n656 = case shown="False" w1680 {
                tunnel: w1685 -> [w1715 _]
                tunnel: w1684 -> [w1714 _]
                tunnel: w1683 -> [w1713 _]
                tunnel: [w1711 w1722] -> w1682
                tunnel: w1681 -> [w1710 w1722]
                frame False {
                  n657 = Unbundle By Name(w1713) -> ("Left"=w1716:i32, "Top"=w1717:i32, "Right"=w1720:i32, "Bottom"=w1712:i32)
                  n658 = In Range and Coerce(upper limit=w1720, x=w1715, lower limit=w1716) -> (In Range?=w1718:bool)  [unwired: 1 out]
                  n659 = In Range and Coerce(upper limit=w1712, x=w1714, lower limit=w1717) -> (In Range?=w1719:bool)  [unwired: 1 out]
                  n660 = And(x=w1718, y=w1719) -> (x .and. y?=w1721:bool)
                  n661 = Select(t=w1710, s=w1721, f=37) -> (s? t:f=w1711:i32)
                }
                frame True {
                  # "Stim path = Imaging path - no bounding box required!"
                }
              }
              n662 = Bundle By Name(cluster=T16 {"ROI name"="", "pixel coordinates"={"x"=0, "y"=0}} ("notebook"), "ROI name"=w1687, "pixel coordinates.x"=w1685, "pixel coordinates.y"=w1684) -> (w1688:T16)
              n663 = Bundle(w1685, w1684) -> (w1679:cluster{i32, i32})  [unwired: 1 in]
              n664 = call "IMAQ Overlay Text"("Group"=w1678, "Text Color (black)"=u32 16711680, "Font, Size & Style"=T28 {"Desired Font (Application)"=enum."Application Font", "[User-specified Font]"={"Font Name"="", "Size"=8, "Strikeout?"=FALSE, "Italic?"=FALSE, "Underline?"=FALSE, "Outline?"=FALSE, "Shadow?"=FALSE, "Bold?"=FALSE, "Rotation Angle"=0.0}, "Horizontal Alignment"=0, "Vertical Alignment"=0}, "String"=w1678, "Origin"=w1679, "Image"=w1677) -> ()  [unwired: 4 in, 2 out]
              n665 = call "IMAQ Convert Point to ROI"("Point"=w1679) -> ("ROI Descriptor"=w1690:T30)  [unwired: 8 in, 1 out]
              n666 = Build Array(w1690) -> (w1696:T30[])
              n667 = call "IMAQ Group ROIs"("ROI Descriptors"=w1696) -> ("ROI Descriptor out"=w1691:T30)  [unwired: 3 in, 1 out]
              n668 = call "IMAQ Overlay ROI"("Colors (Green)"=u32[] [16716800], "Group"=w1678, "Point Symbol"=u32[][] [[16777216, 16777216, 16777216, 1689600, 16777216, 16777216, 16777216], [16777216, 16777216, 16777216, 51267, 16777216, 16777216, 16777216], [16777216, 16777216, 16777216, 1703680, 16777216, 16777216, 16777216], [56363, 65316, 65316, 65316, 1244955, 65351, 711680], [16777216, 16777216, 16777216, 65351, 16777216, 16777216, 16777216], [16777216, 16777216, 16777216, 1244955, 16777216, 16777216, 16777216], [16777216, 16777216, 16777216, 1244955, 16777216, 16777216, 16777216]], "ROI Descriptor"=w1691, "Image"=w1677) -> ("Image Out"=w1686:T1)  [unwired: 5 in, 1 out]
            }
            n669 = Decrement(x=w1643) -> (x-1=w1642:i32)
            n670 = call "No color_Stim Prot.vi"("Protocol Editor reference IN"=w1636) -> ("error out"=w1635:errorcluster, "Protocol Editor reference OUT"=w1634:refnum<vi>)  [unwired: 9 in]
            n671 = Close Reference(reference=w1634, error in (no error)=w1635) -> (error out=w1633:errorcluster)
            n672 = Array Subset "All columns, but not the first"(array=w1646, index (col)=1 ("index"), length (col)=w1642) -> (w1641:string[][])  [unwired: 2 in]
            n673 = for "Check for invaild cells, set BG color accordingly" {
              tunnel: w1641 -> [w1666] mode=indexing
              tunnel: [w1664] -> w1640 mode=concatenating
              tunnel: w1633 -> [_]
              i -> [w1665]
              n674 = for {
                tunnel: w1666 -> [w1676] mode=indexing
                tunnel: w1665 -> [w1669]
                tunnel: [w1671] -> w1664 mode=indexing if=w1670
                i -> [w1668]
                n675 = Increment(x=w1668) -> (x+1=w1667:i32)
                n676 = Bundle By Name(cluster=T6 {"Row"=0, "Column"=0} ("Active Cell:Active Cell"), "Row"=w1669, "Column"=w1667) -> (w1671:T6)
                n677 = call "string test_single_cell.vi"("Column"=w1667, "string"=w1676) -> ("String invalid!"=w1670:bool)  [unwired: 8 in]
                n678 = Select(t=u32 15663114, s=w1670, f=u32 16777226) -> (s? t:f=w1673:u32)
                n679 = property on="Protocol Editor" class="MCListbox (strict)"("ActiveCell"=w1671, "CellBG"=w1673) -> ()  [unwired: 2 in, 2 out]
              }
            }
            n680 = global write "save ROI.vi" "Save Coordinates"(w1639) -> ()
            n681 = call "IMAQ Copy Overlay"("Image Dst"=w1621, "Image Src"=w1622) -> ("Image Dst Out"=w1627:T1)  [unwired: 8 in, 1 out]
            n682 = call "IMAQ Copy Overlay"("Image Dst"=w1627, "Image Src"=w1628) -> ()  [unwired: 8 in, 2 out]
            n683 = property on="Protocol Editor" class="MCListbox (strict)"("ItemNames"=w1646, "ItemSyms"=w1629) -> ()  [unwired: 2 in, 2 out]
          }
          frame True {
          }
        }
      }
      event "Imaging Shutter": Value Change {
        n684 = event-data() -> ("NewVal"=w1736:bool)  [unwired: 1 in]
        n685 = call-poly "GFGpolyGet.vi"("Variable Name in"="scanner.type") -> ("String"=w1733:string)  [unwired: 9 in, 1 out]
        n686 = case shown="\"Imaging Path Galvo\", \"Imaging Path Reso\"" w1733 {
          tunnel: w1736 -> [_ w1743]
          frame Default {
          }
          frame "Imaging Path Galvo", "Imaging Path Reso" {
            # "Update Shutter in  the Main SciScan UI"
            n687 = call "GFG_core.vi"("Variable Name in"="shutter", "Variant in"=w1743, "Action"=enum16{"Init", "Set", "Get", "Clear"}."Set") -> ()  [unwired: 10 in, 7 out]
          }
        }
        n688 = call "GFG_core.vi"("Variable Name in"="Imaging.Shutter", "Variant in"=w1736, "Action"=enum16{"Init", "Set", "Get", "Clear"}."Set") -> ()  [unwired: 10 in, 7 out]
      }
      event "Reverse": Value Change {
        # "Redraw whole list white"
        # "Invert the list"
        n689 = event-data() -> ()  [unwired: 1 in, 1 out]
        n690 = property class="MCListbox (strict)"(reference=w1766) -> (reference out=w1761:refnum<vi>, error out=w1760:errorcluster, "ItemNames"=w1765:string[][], "ItemSyms"=w1763:i32[])  [unwired: 1 in]
        n691 = case shown="True" w1771 {
          tunnel: [w1805 FALSE ("Waveform changed!")] -> w1770
          frame False {
            w1805 = TRUE  # Waveform changed!
          }
          frame True {
            n692 = property on="Update waveform and Timing" class="Bool (strict)"("Val(Sgnl)"=TRUE ("Value (Signaling)")) -> ()  [unwired: 2 in, 2 out]
          }
        }
        n693 = Transpose 2D Array(2D array=w1765) -> (transposed array=w1764:string[][])
        n694 = for {
          tunnel: w1764 -> [w1804] mode=indexing
          tunnel: [w1803] -> w1762 mode=indexing
          n695 = Reverse 1D Array(array=w1804) -> (reversed array=w1803:string[])
        }
        n696 = Reverse 1D Array(array=w1763) -> (reversed array=w1759:i32[])
        n697 = Transpose 2D Array(2D array=w1762) -> (transposed array=w1757:string[][])
        n698 = property class="MCListbox (strict)"(reference=w1761, error in=w1760, "ItemNames"=w1757, "ItemSyms"=w1759) -> (reference out=w1758:refnum<vi>, error out=w1756:errorcluster)
        n699 = call "No color_Stim Prot.vi"("error in (no error)"=w1756, "Protocol Editor reference IN"=w1758) -> ("error out"=w1754:errorcluster, "Protocol Editor reference OUT"=w1755:refnum<vi>)  [unwired: 8 in]
        n700 = Empty Array?(array=w1750) -> (empty?=w1749:bool)
        n701 = case shown="False" w1749 {
          tunnel: w1757 -> [w1788 _]
          tunnel: w1755 -> [w1784 w1802]
          tunnel: w1754 -> [w1783 w1801]
          tunnel: [w1782 w1800] -> w1753
          tunnel: [w1781 w1801] -> w1752
          tunnel: [w1780 w1802] -> w1751
          tunnel: w1750 -> [w1778 w1800]
          frame False {
            # "Update the list of invalid cells so that the order is correct!"
            n702 = Array Size(array=w1788) -> (size(s)=w1787:i32[])
            n703 = Index Array "# Rows"(array=w1787, index=0) -> (element=w1779:i32)
            n704 = Decrement(x=w1779) -> (x-1=w1785:i32)
            n705 = for {
              tunnel: w1778 -> [w1797] mode=indexing
              tunnel: w1785 -> [w1799]
              tunnel: [w1795] -> w1782 mode=indexing
              n706 = Unbundle By Name(w1797) -> ("Row"=w1798:i32)
              n707 = Subtract(x=w1799, y=w1798) -> (x-y=w1796:i32)
              n708 = Bundle By Name(cluster=w1797, "Row"=w1796) -> (w1795:T6)
            }
            n709 = for "Redraw invaild cells red" {
              tunnel: w1784 -> [w1794]
              tunnel: w1783 -> [w1793]
              tunnel: w1782 -> [w1791] mode=indexing
              tunnel: [w1790] -> w1780
              tunnel: [w1789] -> w1781
              n710 = property class="MCListbox (strict)"(reference=w1794, error in=w1793, "ActiveCell"=w1791, "CellBG"=u32 16711680) -> (reference out=w1790:refnum<vi>, error out=w1789:errorcluster)
            }
          }
          frame True {
          }
        }
        n711 = Close Reference(reference=w1751, error in (no error)=w1752) -> ()  [unwired: 1 out]
      }
      event "random": Value Change {
        n712 = event-data() -> ()  [unwired: 1 in, 1 out]
        n713 = case shown="True" w1837 {
          tunnel: [w1857 FALSE ("Waveform changed!")] -> w1836
          frame False {
            w1857 = TRUE  # Waveform changed!
          }
          frame True {
            n714 = property on="Update waveform and Timing" class="Bool (strict)"("Val(Sgnl)"=TRUE ("Value (Signaling)")) -> ()  [unwired: 2 in, 2 out]
          }
        }
        n715 = property on="Property Node" class="MCListbox (strict)"(reference=w1823) -> (reference out=w1818:refnum<vi>, error out=w1817:errorcluster, "ItemNames"=w1822:string[][], "ItemSyms"=w1821:i32[])  [unwired: 1 in]
        n716 = Array Size(array=w1822) -> (size(s)=w1826:i32[])
        n717 = Index Array(array=w1826, index=0) -> (element=w1824:i32)
        n718 = for "Randomise order" {
          N: w1824 -> [_]
          shift-right: [w1866] -> w1819
          shift-left: w1822 -> [w1869]
          shift-right: [w1860] -> w1820
          shift-left: w1821 -> [w1864]
          i -> [w1865]
          n719 = Random Number (0-1)() -> (number: 0 to 1=w1872:dbl)
          n720 = Multiply(x=w1865, y=w1872) -> (x*y=w1871:dbl)
          n721 = Round To Nearest(number=w1871) -> (nearest integer value=w1870:dbl)
          n722 = To Long Integer(number=w1870) -> (32bit integer=w1863:i32)
          n723 = Delete From Array(array=w1869, index (row)=w1863) -> (deleted portion=w1867:string[], array with subset deleted=w1868:string[][])  [unwired: 2 in]
          n724 = Delete From Array(array=w1864, index=w1863) -> (deleted portion=w1861:i32, array with subset deleted=w1862:i32[])  [unwired: 1 in]
          n725 = Insert Into Array(array=w1868, new element=w1867) -> (w1866:string[][])  [unwired: 2 in]
          n726 = Insert Into Array(array=w1862, new element=w1861) -> (w1860:i32[])  [unwired: 1 in]
        }
        n727 = property on="Property Node" class="MCListbox (strict)"(reference=w1818, error in=w1817, "ItemNames"=w1819, "ItemSyms"=w1820) -> (reference out=w1816:refnum<vi>, error out=w1815:errorcluster)
        n728 = Array Size(array=w1819) -> (size(s)=w1831:i32[])
        n729 = Index Array(array=w1831, index=1) -> (element=w1829:i32)
        n730 = Decrement(x=w1829) -> (x-1=w1828:i32)
        n731 = call "No color_Stim Prot.vi"("error in (no error)"=w1815, "Protocol Editor reference IN"=w1816) -> ("error out"=w1813:errorcluster, "Protocol Editor reference OUT"=w1814:refnum<vi>)  [unwired: 8 in]
        n732 = Close Reference(reference=w1814, error in (no error)=w1813) -> (error out=w1812:errorcluster)
        n733 = Array Subset "All columns, but not the first"(array=w1819, index (col)=1 ("index"), length (col)=w1828) -> (w1827:string[][])  [unwired: 2 in]
        n734 = for "Check for invaild cells, set BG color accordingly" {
          tunnel: w1827 -> [w1846] mode=indexing
          tunnel: [w1844] -> w1811 mode=concatenating
          tunnel: w1812 -> [_]
          i -> [w1845]
          n735 = for {
            tunnel: w1846 -> [w1856] mode=indexing
            tunnel: w1845 -> [w1849]
            tunnel: [w1851] -> w1844 mode=indexing if=w1850
            i -> [w1848]
            n736 = Increment(x=w1848) -> (x+1=w1847:i32)
            n737 = Bundle By Name(cluster=T6 {"Row"=0, "Column"=0} ("Active Cell:Active Cell"), "Row"=w1849, "Column"=w1847) -> (w1851:T6)
            n738 = call "string test_single_cell.vi"("Column"=w1847, "string"=w1856) -> ("String invalid!"=w1850:bool)  [unwired: 8 in]
            n739 = Select(t=u32 15663114, s=w1850, f=u32 16777226) -> (s? t:f=w1853:u32)
            n740 = property on="Protocol Editor" class="MCListbox (strict)"("ActiveCell"=w1851, "CellBG"=w1853) -> ()  [unwired: 2 in, 2 out]
          }
        }
      }
      event "Delete": Value Change {
        n741 = event-data() -> ()  [unwired: 1 in, 1 out]
        n742 = property on="Protocol Editor" class="MCListbox (strict)"() -> ("ItemNames"=w1896:string[][], "Value"=w1895:i32[])  [unwired: 2 in, 2 out]
        n743 = property on="Protocol Editor" class="MCListbox (strict)"() -> ("ItemSyms"=w1890:i32[])  [unwired: 2 in, 2 out]
        n744 = Empty Array?(array=w1895) -> (empty?=w1894:bool)
        n745 = case shown="False" w1894 {
          tunnel: w1896 -> [w1915 _]
          tunnel: w1895 -> [w1924 _]
          tunnel: w1888 -> [w1914 _]
          tunnel: w1890 -> [w1917 _]
          tunnel: w1887 -> [w1910 _]
          tunnel: [w1911 w1986] -> w1884
          tunnel: w1883 -> [_ w1986]
          tunnel: w1882 -> [w1912 _]
          tunnel: w1878 -> [w1898 w1985]
          tunnel: [w1897 w1984] -> w1877
          tunnel: w1876 -> [_ w1984]
          frame False {
            w1913 = string[] []  # Remaining Groups
            n746 = Sort 1D Array(array=w1924) -> (sorted array=w1927:i32[])
            n747 = Build Array (concatenate)(-1 ("Numeric"), w1927) -> (w1925:i32[])
            n748 = case shown="True" w1912 {
              tunnel: [w1948 FALSE ("Waveform changed!")] -> w1911
              frame False {
                w1948 = TRUE  # Waveform changed!
              }
              frame True {
                n749 = property on="Update waveform and Timing" class="Bool (strict)"("Val(Sgnl)"=TRUE ("Value (Signaling)")) -> ()  [unwired: 2 in, 2 out]
              }
            }
            n750 = for {
              tunnel: w1927 -> [w1962] mode=indexing
              tunnel: w1925 -> [w1961] mode=indexing
              tunnel: [w1960] -> w1930 mode=indexing
              n751 = Not Equal?(x=w1962, y=w1961) -> (x != y?=w1960:bool)
            }
            n752 = call "array to filter array.vi"("keep elements?"=w1930) -> ("insertion list"=w1929:i32[])  [unwired: 4 in]
            n753 = for {
              tunnel: w1927 -> [w1959]
              tunnel: w1929 -> [w1958] mode=indexing
              tunnel: [w1957] -> w1928 mode=indexing
              n754 = Index Array(array=w1959, index=w1958) -> (element=w1957:i32)
            }
            n755 = Reverse 1D Array(array=w1928) -> (reversed array=w1931:i32[])
            n756 = for {
              shift-right: [w1967] -> w1923
              shift-left: w1915 -> [w1968]
              tunnel: w1931 -> [w1965] mode=indexing
              tunnel: [w1966] -> w1922 mode=indexing
              shift-right: [w1963] -> w1916
              shift-left: w1917 -> [w1964]
              n757 = Delete From Array(array=w1964, index=w1965) -> (array with subset deleted=w1963:i32[])  [unwired: 1 in, 1 out]
              n758 = Delete From Array(array=w1968, index (row)=w1965) -> (deleted portion=w1966:string[], array with subset deleted=w1967:string[][])  [unwired: 2 in]
            }
            n759 = global read "save ROI.vi" "Save Coordinates"() -> (w1934:T10)
            n760 = Index Array(array=w1923, index (col)=0 ("disabled index (col)")) -> (element=w1932:string[])  [unwired: 1 in]
            n761 = Index Array(array=w1922, index (col)=0 ("disabled index (col)")) -> (element=w1920:string[])  [unwired: 1 in]
            n762 = call "save coor order.vi"("Save Coordinates"=w1934, "Stm ID"=w1932) -> ()  [unwired: 9 in, 1 out]
            n763 = for {
              tunnel: w1920 -> [w1955] mode=indexing
              tunnel: [w1954] -> w1918 mode=indexing
              n764 = Search/Split String(string=w1955, search string/char (-)="[" ("regular expression")) -> (substring before match=w1954:string)  [unwired: 1 in, 2 out]
            }
            n765 = for {
              tunnel: w1918 -> [w1973] mode=indexing
              shift-right: [w1974] -> w1909
              shift-left: string[] [] -> [w1975]
              shift-right: [w1969] -> _
              shift-left: w1913 -> [w1970]
              n766 = Equal?(x=w1973, y="") -> (x = y?=w1972:bool)
              n767 = case "If \"F\" then add row to results." shown="False" w1972 {
                tunnel: w1975 -> [w1979 w1983]
                tunnel: w1973 -> [w1978 w1981]
                tunnel: [w1977 w1983] -> w1974
                tunnel: w1970 -> [w1976 w1982]
                tunnel: [w1976 w1980] -> w1969
                frame False {
                  n768 = Insert Into Array(array=w1979, new element=w1978) -> (w1977:string[])  [unwired: 1 in]
                }
                frame True {
                  n769 = Insert Into Array(array=w1982, new element=w1981) -> (w1980:string[])  [unwired: 1 in]
                }
              }
            }
            n770 = Array Size(array=w1899) -> (size(s)=w1901:i32[])
            n771 = Index Array(array=w1901, index=1) -> (element=w1903:i32)
            n772 = Decrement(x=w1903) -> (x-1=w1904:i32)
            n773 = call "No color_Stim Prot.vi"("Protocol Editor reference IN"=w1898) -> ("error out"=w1907:errorcluster, "Protocol Editor reference OUT"=w1906:refnum<vi>)  [unwired: 9 in]
            n774 = Close Reference(reference=w1906, error in (no error)=w1907) -> (error out=w1908:errorcluster)
            n775 = Array Subset "All columns, but not the first"(array=w1899, index (col)=1 ("index"), length (col)=w1904) -> (w1905:string[][])  [unwired: 2 in]
            n776 = for "Check for invaild cells, set BG color accordingly" {
              tunnel: w1905 -> [w1937] mode=indexing
              tunnel: [w1935] -> w1897 mode=concatenating
              tunnel: w1908 -> [_]
              i -> [w1936]
              n777 = for {
                tunnel: w1937 -> [w1947] mode=indexing
                tunnel: w1936 -> [w1940]
                tunnel: [w1942] -> w1935 mode=indexing if=w1941
                i -> [w1939]
                n778 = Increment(x=w1939) -> (x+1=w1938:i32)
                n779 = Bundle By Name(cluster=T6 {"Row"=0, "Column"=0} ("Active Cell:Active Cell"), "Row"=w1940, "Column"=w1938) -> (w1942:T6)
                n780 = call "string test_single_cell.vi"("Column"=w1938, "string"=w1947) -> ("String invalid!"=w1941:bool)  [unwired: 8 in]
                n781 = Select(t=u32 15663114, s=w1941, f=u32 16777226) -> (s? t:f=w1944:u32)
                n782 = property on="Protocol Editor" class="MCListbox (strict)"("ActiveCell"=w1942, "CellBG"=w1944) -> ()  [unwired: 2 in, 2 out]
              }
            }
            n783 = call "IMAQ Clear Overlay"("Groups"=w1909, "Image"=w1914) -> ()  [unwired: 8 in, 2 out]
            n784 = call "IMAQ Clear Overlay"("Groups"=w1909, "Image"=w1910) -> ()  [unwired: 8 in, 2 out]
            n785 = flat-sequence {
              tunnel: w1923 -> [w1951]
              tunnel: w1916 -> [w1952]
              tunnel: w1909 -> [_]
              tunnel: [w1951] -> w1899
              frame #0 {
                n786 = property on="Protocol Editor" class="MCListbox (strict)"("ItemNames"=w1951, "Value"=i32[] [] ("Stimulation Protocol"), "ItemSyms"=w1952) -> ()  [unwired: 2 in, 2 out]
              }
            }
          }
          frame True {
            n787 = Close Reference(reference=w1985) -> ()  [unwired: 1 in, 1 out]
            n788 = One Button Dialog(message="Please select the row to delete.") -> ()  [unwired: 1 in, 1 out]
          }
        }
      }
      event Value Change {
        n789 = event-data() -> ()  [unwired: 1 in, 1 out]
        n790 = call <vilib>:"Application Directory.vi"() -> ("Application Directory"=w2000:path)
        n791 = Build Path(base path=w2000, name or relative path="Parallel Uncaging Module\\Calibration_GUI.vi") -> (appended path=w1998:path)
        n792 = Open VI Reference(vi path=w1998) -> (vi reference=w2007:refnum<vi>)  [unwired: 5 in, 1 out]
        n793 = invoke class="VI" method="FP.Open"(reference=w2007) -> (reference out=w2006:refnum<vi>, error out=w2005:errorcluster)  [unwired: 4 in, 3 out]
        n794 = invoke class="VI" method="Run VI"(reference=w2006, error in=w2005, "Wait until done"=FALSE ("Wait Until Done")) -> (reference out=w2003:refnum<vi>, error out=w2002:errorcluster)  [unwired: 2 in, 3 out]
        n795 = Close Reference(reference=w2003, error in (no error)=w2002) -> (error out=w2001:errorcluster)
        n796 = call <vilib>:"Clear Errors.vi"("error in (no error)"=w2001) -> ()  [unwired: 6 in, 1 out]
      }
      event "Pre-stim baseline (s)", "Pre-Stim Baseline", "Rep interval (s)", "Group reps": Value Change {
        n797 = event-data() -> ()  [unwired: 1 in, 1 out]
        n798 = case shown="True" w2020 {
          tunnel: [w2027 FALSE ("Waveform changed!")] -> w2019
          frame False {
            w2027 = TRUE  # Waveform changed!
          }
          frame True {
            n799 = property on="Update waveform and Timing" class="Bool (strict)"("Val(Sgnl)"=TRUE ("Value (Signaling)")) -> ()  [unwired: 2 in, 2 out]
          }
        }
      }
      event "stop": Value Change {
        n800 = event-data() -> ()  [unwired: 1 in, 1 out]
      }
      event Panel Close? {
        n801 = event-data() -> ()  [unwired: 1 in, 1 out]
        n802 = control-ref of="This VI"() -> (w2058:refnum<vi>)
        n803 = property class="VI"(reference=w2058, "FP.State"=T29."Hidden" ("Front Panel Window:State")) -> (reference out=w2056:refnum<vi>, error out=w2057:errorcluster)  [unwired: 1 in]
        n804 = Close Reference(reference=w2056, error in (no error)=w2057) -> ()  [unwired: 1 out]
        n805 = event-data("Discard?"=TRUE) -> ()  [unwired: 1 in, 1 out]
      }
    }
    "Image1" <- w140
  }
